vi "Text control 2 v6.4_pump-specific.vi"() -> ()   [LabVIEW 2016]
panel:
  in  "Tab Control":enum32{"Main", "Other parameters"}(tab)
  out "Line running":i32
  out "Total lines":i32
  out "Path":path=path "C:/users/rlp38/09Apr2009LTtesting/test2.txt"
  out "I vs Vg":cluster{"Y data in":dbl[], "X data in":dbl[]}[](graph)
  out "Is max":dbl format="%.2e"
  out "Id max":dbl format="%.2e"
  out "Ig max":dbl format="%.2e"
  out "Imax vs time":cluster{"Y data in":dbl[], "X data in":dbl[]}[](graph)
  out "Imin vs time":cluster{"Y data in":dbl[], "X data in":dbl[]}[](graph)
  out "I vs Vd":cluster{"Y data in":dbl[], "X data in":dbl[]}[](graph)
  in  "Script":string="#-------------------------------------------------------\n# SPM pump cleaning script\n#\n# Version: 0.5\n# Author: Dimitrios Simatos\n# Last updated: 2018-01-05\n#-------------------------------------------------------\n# Description\n#\n# This script is designed to run the cleaning sequence of the SPM OEM pump.\n# This script needs to be run 4 times!\n#-------------------------------------------------------\n# Changes\n#\n# Placed initialization and hard stop commands in the beginning.\n#-------------------------------------------------------\n# Important points\n#\n# Never leave any liquid in the pump to dry after the experiments. If they dry, the residue may block the valve.\n# Always run the cleaning cycle after the experiments.\n# Use clockwise rotation when going up in valve port numbers and vice versa.\n#-------------------------------------------------------\n# Things to do before running the script\n#\n# Set time units to minutes.\n# Set filenames.\n# Replace the tubing, if necessary.\n#-------------------------------------------------------\n# Port connections\n#\n# Port 1: Waste\n# Port 2: Waste\n# Port 3: Various cleaning liquids\n# Port 4: Waste\n# Port 5: Waste\n# Port 6: Waste\n#\n# Between each of the 4 runs, the settings of Port 3 will change, according to the cleaning protocol.\n# The settings for Port 3 are:\n# 1st run: 1% v/v solution of sodium hypochlorite in ultrapure water\n# 2nd run: 0.1% w/v solution of sodium dodecyl sulfate in ultrapure water\n# 3rd run: Ultrapure water\n# 4th run: Waste (in air, not immersed in liquid)\n#-------------------------------------------------------\n# Cleaning protocol for the SPM OEM pump (from the manual)\n#\n# A cleaning procedure should be performed at the end of each day or in between two different experiments.\n# An effective cleaning can be performed in the following manner:\n# • Bleach solution to kill microorganisms\n# 1. Prepare a solution of 1% chlorine bleach and deionized water\n#    NOTE: Prepare a 1% v/v solution of sodium hypochlorite in deionized water\n# 2. Prepare a reservoir and place 1 tubing in the bleach solution and 5 tubings in a waste recipient\n# 3. Pick up the bleach solution through 1 port to entirely fill the syringe\n# 4. Sequentially output the syringe content through the remaining ports and throw it to the waste\n# 5. Repeat operation at least 2 times\n# • Detergent solution to remove debris\n# 1. Prepare a solution of 0.1% detergent and deionized water\n#    NOTE: Prepare a 0.1% w/v solution of sodium dodecyl sulfate in deionized water\n# 2. Move the tubing from the bleach solution reservoir and place it into a reservoir of detergent solution\n# 3. Pick up the detergent solution through 1 port to entirely fill the syringe\n# 4. Sequentially output the detergent solution through the remaining ports into the waste recipient\n# 5. Repeat operation at least 2 times\n# • Rinsing water to prepare the pump for your next experiment\n# 1. Move the tubing from the detergent solution reservoir and place it into a reservoir of deionized water\n# 2. Pick up the rinsing solution through 1 port to entirely fill the syringe\n# 3. Sequentially output the rinse water through the remaining ports into the waste recipient\n# 4. Repeat operation at least 2 times\n# • Replace the tubing, if necessary\n#-------------------------------------------------------\n# Pumping cycles and execution time\n#\n# Execution time for a single cycle: 6 x (1 min + 10 sec) = 7 minutes\n# Total execution time: 4 x 7 = 28 minutes\n# Since the script has to run 4 times, the cleaning lasts for: 4 x 28 = 112 minutes\n# Air must be the last to be pumped through the valve, to remove all liquids.\n# There are 4 pumping cycles. Each one draws a different liquid through port 3 and pumps it sequentially through ports 1,2,4,5,6.\n# During the sequential pumping, each port receives 200 ml of liquid (20% of the total syringe volume = 600 \"plunger units\")\n# The device must be disconnected from the port during the cleaning procedure.\n# All cycles are similar, except cycle 1 has the initialization command uncommented and the first report valve command commented.\n#-------------------------------------------------------\n# Volume of liquid needed\n#\n# Volume of liquid needed per cycle: 1 ml\n# Total volume of liquid needed per script run: 4 x 1 = 4 ml\n# Since the script has to run 4 times, the first 3 with different liquids, I need:\n# 4 ml of 1% v/v solution of sodium hypochlorite in ultrapure water\n# 4 ml of 0.1% w/v solution of sodium dodecyl sulfate in ultrapure water\n# 4 ml of ultrapure water\n#-------------------------------------------------------\n# Parameters\n#\n# Syringe size: 1 ml\n# Step resolution N = 0.01 mm\n# Drawing flow V = 300 pulses/second (6000 ul/min)\n# Pumping flow V = 300 pulses/second (6000 ul/min)\n#-------------------------------------------------------\n# Pump initialization\npump /1T #hard stop pump\npump /1ZR #initialize pump\n#-------------------------------------------------------\n# Cycle 1\n# Fill the syringe\npump /1Q #query pump\npump /1? #report absolute plunger position\n#pump /1?6 #report valve position\nwait-min 1 #wait 1 minute\npump /1N0R #set step resolution: 0.01 mm\npump /1Q #query pump\npump /1? #report absolute plunger position (the plunger should be at 0)\npump /1?6 #report valve position\nwait 1000 #wait 1 second\npump /1V300R #choose speed: 300 steps/s (6000 ul/min)\npump /1Q #query pump\nwait 1000 #wait 1 second\npump /1I3R #go to port 3, clockwise rotation\npump /1Q #query pump\npump /1?6 #report valve position\nwait 1000 #wait 1 second\npump /1A3000R #go to absolute position 3000 (= draw 1 ml)\nwait 30000 #wait 30 seconds\npump /1Q #query pump\npump /1? #report absolute plunger position (the plunger should have finished moving)\n#pump /1?6 #report valve position\n# The sequential pumping begins\n# Port 1\npump /1O1R #switch to port 1, counterclockwise rotation\npump /1Q #query pump\npump /1?6 #report valve position\npump /1A2400R #go to absolute position 2400 (= pump 200 ul)\npump /1Q #query pump\npump /1? #report absolute plunger position (the plunger should be moving to 0)\nwait-min 1 #wait 1 minute\npump /1? #report absolute plunger position (the plunger should have finished moving)\n# Port 2\npump /1I2R #switch to port 2, clockwise rotation\npump /1Q #query pump\npump /1?6 #report valve position\npump /1A1800R #go to absolute position 1800 (= pump 200 ul)\npump /1Q #query pump\npump /1? #report absolute plunger position (the plunger should be moving to 0)\nwait-min 1 #wait 1 minute\npump /1? #report absolute plunger position (the plunger should have finished moving)\n# Port 4\npump /1I4R #switch to port 4, clockwise rotation\npump /1Q #query pump\npump /1?6 #report valve position\npump /1A1200R #go to absolute position 1200 (= pump 200 ul)\npump /1Q #query pump\npump /1? #report absolute plunger position (the plunger should be moving to 0)\nwait-min 1 #wait 1 minute\npump /1? #report absolute plunger position (the plunger should have finished moving)\n# Port 5\npump /1I5R #switch to port 5, clockwise rotation\npump /1Q #query pump\npump /1?6 #report valve position\npump /1A600R #go to absolute position 600 (= pump 200 ul)\npump /1Q #query pump\npump /1? #report absolute plunger position (the plunger should be moving to 0)\nwait-min 1 #wait 1 minute\npump /1? #report absolute plunger position (the plunger should have finished moving)\n# Port 6\npump /1I6R #switch to port 6, clockwise rotation\npump /1Q #query pump\npump /1?6 #report valve position\npump /1A0R #go to absolute position 0 (= pump 200 ul)\npump /1Q #query pump\npump /1? #report absolute plunger position (the plunger should be moving to 0)\nwait-min 1 #wait 1 minute\npump /1? #report absolute plunger position (the plunger should have finished moving)\n#-------------------------------------------------------\n# Cycle 2\n# Fill the syringe\n#pump /1ZR #initialize pump\npump /1Q #query pump\npump /1? #report absolute plunger position\npump /1?6 #report valve position\nwait-min 1 #wait 1 minute\npump /1N0R #set step resolution: 0.01 mm\npump /1Q #query pump\npump /1? #report absolute plunger position (the plunger should be at 0)\npump /1?6 #report valve position\nwait 1000 #wait 1 second\npump /1V300R #choose speed: 300 steps/s (6000 ul/min)\npump /1Q #query pump\nwait 1000 #wait 1 second\npump /1O3R #go to port 3, counterclockwise rotation\npump /1Q #query pump\npump /1?6 #report valve position\nwait 1000 #wait 1 second\npump /1A3000R #go to absolute position 3000 (= draw 1 ml)\nwait 30000 #wait 30 seconds\npump /1Q #query pump\npump /1? #report absolute plunger position (the plunger should have finished moving)\n#pump /1?6 #report valve position\n# The sequential pumping begins\n# Port 1\npump /1O1R #switch to port 1, counterclockwise rotation\npump /1Q #query pump\npump /1?6 #report valve position\npump /1A2400R #go to absolute position 2400 (= pump 200 ul)\npump /1Q #query pump\npump /1? #report absolute plunger position (the plunger should be moving to 0)\nwait-min 1 #wait 1 minute\npump /1? #report absolute plunger position (the plunger should have finished moving)\n# Port 2\npump /1I2R #switch to port 2, clockwise rotation\npump /1Q #query pump\npump /1?6 #report valve position\npump /1A1800R #go to absolute position 1800 (= pump 200 ul)\npump /1Q #query pump\npump /1? #report absolute plunger position (the plunger should be moving to 0)\nwait-min 1 #wait 1 minute\npump /1? #report absolute plunger position (the plunger should have finished moving)\n# Port 4\npump /1I4R #switch to port 4, clockwise rotation\npump /1Q #query pump\npump /1?6 #report valve position\npump /1A1200R #go to absolute position 1200 (= pump 200 ul)\npump /1Q #query pump\npump /1? #report absolute plunger position (the plunger should be moving to 0)\nwait-min 1 #wait 1 minute\npump /1? #report absolute plunger position (the plunger should have finished moving)\n# Port 5\npump /1I5R #switch to port 5, clockwise rotation\npump /1Q #query pump\npump /1?6 #report valve position\npump /1A600R #go to absolute position 600 (= pump 200 ul)\npump /1Q #query pump\npump /1? #report absolute plunger position (the plunger should be moving to 0)\nwait-min 1 #wait 1 minute\npump /1? #report absolute plunger position (the plunger should have finished moving)\n# Port 6\npump /1I6R #switch to port 6, clockwise rotation\npump /1Q #query pump\npump /1?6 #report valve position\npump /1A0R #go to absolute position 0 (= pump 200 ul)\npump /1Q #query pump\npump /1? #report absolute plunger position (the plunger should be moving to 0)\nwait-min 1 #wait 1 minute\npump /1? #report absolute plunger position (the plunger should have finished moving)\n#-------------------------------------------------------\n# Cycle 3\n# Fill the syringe\n#pump /1ZR #initialize pump\npump /1Q #query pump\npump /1? #report absolute plunger position\npump /1?6 #report valve position\nwait-min 1 #wait 1 minute\npump /1N0R #set step resolution: 0.01 mm\npump /1Q #query pump\npump /1? #report absolute plunger position (the plunger should be at 0)\npump /1?6 #report valve position\nwait 1000 #wait 1 second\npump /1V300R #choose speed: 300 steps/s (6000 ul/min)\npump /1Q #query pump\nwait 1000 #wait 1 second\npump /1O3R #go to port 3, counterclockwise rotation\npump /1Q #query pump\npump /1?6 #report valve position\nwait 1000 #wait 1 second\npump /1A3000R #go to absolute position 3000 (= draw 1 ml)\nwait 30000 #wait 30 seconds\npump /1Q #query pump\npump /1? #report absolute plunger position (the plunger should have finished moving)\n#pump /1?6 #report valve position\n# The sequential pumping begins\n# Port 1\npump /1O1R #switch to port 1, counterclockwise rotation\npump /1Q #query pump\npump /1?6 #report valve position\npump /1A2400R #go to absolute position 2400 (= pump 200 ul)\npump /1Q #query pump\npump /1? #report absolute plunger position (the plunger should be moving to 0)\nwait-min 1 #wait 1 minute\npump /1? #report absolute plunger position (the plunger should have finished moving)\n# Port 2\npump /1I2R #switch to port 2, clockwise rotation\npump /1Q #query pump\npump /1?6 #report valve position\npump /1A1800R #go to absolute position 1800 (= pump 200 ul)\npump /1Q #query pump\npump /1? #report absolute plunger position (the plunger should be moving to 0)\nwait-min 1 #wait 1 minute\npump /1? #report absolute plunger position (the plunger should have finished moving)\n# Port 4\npump /1I4R #switch to port 4, clockwise rotation\npump /1Q #query pump\npump /1?6 #report valve position\npump /1A1200R #go to absolute position 1200 (= pump 200 ul)\npump /1Q #query pump\npump /1? #report absolute plunger position (the plunger should be moving to 0)\nwait-min 1 #wait 1 minute\npump /1? #report absolute plunger position (the plunger should have finished moving)\n# Port 5\npump /1I5R #switch to port 5, clockwise rotation\npump /1Q #query pump\npump /1?6 #report valve position\npump /1A600R #go to absolute position 600 (= pump 200 ul)\npump /1Q #query pump\npump /1? #report absolute plunger position (the plunger should be moving to 0)\nwait-min 1 #wait 1 minute\npump /1? #report absolute plunger position (the plunger should have finished moving)\n# Port 6\npump /1I6R #switch to port 6, clockwise rotation\npump /1Q #query pump\npump /1?6 #report valve position\npump /1A0R #go to absolute position 0 (= pump 200 ul)\npump /1Q #query pump\npump /1? #report absolute plunger position (the plunger should be moving to 0)\nwait-min 1 #wait 1 minute\npump /1? #report absolute plunger position (the plunger should have finished moving)\n#-------------------------------------------------------\n# Cycle 4\n# Fill the syringe\n#pump /1ZR #initialize pump\npump /1Q #query pump\npump /1? #report absolute plunger position\npump /1?6 #report valve position\nwait-min 1 #wait 1 minute\npump /1N0R #set step resolution: 0.01 mm\npump /1Q #query pump\npump /1? #report absolute plunger position (the plunger should be at 0)\npump /1?6 #report valve position\nwait 1000 #wait 1 second\npump /1V300R #choose speed: 300 steps/s (6000 ul/min)\npump /1Q #query pump\nwait 1000 #wait 1 second\npump /1O3R #go to port 3, counterclockwise rotation\npump /1Q #query pump\npump /1?6 #report valve position\nwait 1000 #wait 1 second\npump /1A3000R #go to absolute position 3000 (= draw 1 ml)\nwait 30000 #wait 30 seconds\npump /1Q #query pump\npump /1? #report absolute plunger position (the plunger should have finished moving)\n#pump /1?6 #report valve position\n# The sequential pumping begins\n# Port 1\npump /1O1R #switch to port 1, counterclockwise rotation\npump /1Q #query pump\npump /1?6 #report valve position\npump /1A2400R #go to absolute position 2400 (= pump 200 ul)\npump /1Q #query pump\npump /1? #report absolute plunger position (the plunger should be moving to 0)\nwait-min 1 #wait 1 minute\npump /1? #report absolute plunger position (the plunger should have finished moving)\n# Port 2\npump /1I2R #switch to port 2, clockwise rotation\npump /1Q #query pump\npump /1?6 #report valve position\npump /1A1800R #go to absolute position 1800 (= pump 200 ul)\npump /1Q #query pump\npump /1? #report absolute plunger position (the plunger should be moving to 0)\nwait-min 1 #wait 1 minute\npump /1? #report absolute plunger position (the plunger should have finished moving)\n# Port 4\npump /1I4R #switch to port 4, clockwise rotation\npump /1Q #query pump\npump /1?6 #report valve position\npump /1A1200R #go to absolute position 1200 (= pump 200 ul)\npump /1Q #query pump\npump /1? #report absolute plunger position (the plunger should be moving to 0)\nwait-min 1 #wait 1 minute\npump /1? #report absolute plunger position (the plunger should have finished moving)\n# Port 5\npump /1I5R #switch to port 5, clockwise rotation\npump /1Q #query pump\npump /1?6 #report valve position\npump /1A600R #go to absolute position 600 (= pump 200 ul)\npump /1Q #query pump\npump /1? #report absolute plunger position (the plunger should be moving to 0)\nwait-min 1 #wait 1 minute\npump /1? #report absolute plunger position (the plunger should have finished moving)\n# Port 6\npump /1I6R #switch to port 6, clockwise rotation\npump /1Q #query pump\npump /1?6 #report valve position\npump /1A0R #go to absolute position 0 (= pump 200 ul)\npump /1Q #query pump\npump /1? #report absolute plunger position (the plunger should be moving to 0)\nwait-min 1 #wait 1 minute\npump /1? #report absolute plunger position (the plunger should have finished moving)\n#-------------------------------------------------------"
  out "Command running:":string
  out "Serial port data":string
  out "Elapsed Time":dbl caption="Elapsed Time (s)"
  in  "Time Units":u16(ring)=1 items=["Seconds", "Minutes", "Hours"]
  in  "Time Offset":dbl caption="Set Start Time (s)"
  in  "Reset":bool
  in  "Auto Reset":bool
  in  "integration time":u32(slide) max=2 step=1 scale=0.0..2.0
  in  "Interrupt scan":bool
  out "Absolute plunger position vs time":cluster{"Y data in":dbl[], "X data in":dbl[]}[](graph)
  out "Valve position vs time":cluster{"Y data in":dbl[], "X data in":dbl[]}[](graph)
  out "Is on":dbl format="%.2e"
  out "Id on":dbl format="%.2e"
  out "Ig on":dbl format="%.2e"
  out "Ion vs time":cluster{"Y data in":dbl[], "X data in":dbl[]}[](graph)
  out "Ioff vs time":cluster{"Y data in":dbl[], "X data in":dbl[]}[](graph)
  out "Ig min":dbl format="%.2e"
  out "Id min":dbl format="%.2e"
  out "Is min":dbl format="%.2e"
  out "Is off":dbl format="%.2e"
  out "Id off":dbl format="%.2e"
  out "Ig off":dbl format="%.2e"
  in  "Integration time (long)":dbl=0.32 min=0.04 max=2.0 step=0.02 format="%.2f"
  in  "Integration time (short)":dbl=0.0019 min=8e-05 max=0.0019 step=8e-05 format="%^.0e"
  in  "Gate: Compliance":dbl=0.001 format="%.8f"
  in  "Drain: Compliance":dbl=0.001 format="%.8f"
  in  "Hard stop pump":bool
  in  "Halt pump":bool
  in  "Interrupt program":bool
  in  "Suffix (script)":string="step_1_up-H2O_initial_script.txt"
  in  "Filename (variable part)":string="step_1_up-H2O_initial_"
  in  "Plot output curve extrema vs time":bool
  in  "Plot transfer curve extrema vs time":bool=TRUE
  in  "Gate Range\nmode":u16(ring) items=["Auto", "Limited", "Fixed"]
  in  "Gate Range":u8(slide)=6 max=11 scale=0.0..11.0
  in  "Source/Drain\nRange mode":u16(ring) items=["Auto", "Limited", "Fixed"]
  in  "Source/Drain Range":u8(slide)=6 max=11 scale=0.0..11.0
  in  "Panel Controls":T1={"Emergency Stop"=refnum, "TransGraph Max"=1e-05, "Text/Graph (text=false)"=TRUE} {"TransGraph Max" format="%.2e"}
  in  "Panel Controls 2":T2={"Emergency Stop"=refnum, "TransGraph Max"=1e-05, "Text/Graph (text=false)"=TRUE, "TransGraph Min"=1e-11} {"TransGraph Min" format="%.2e"; "TransGraph Max" format="%.2e"}
  in  "SMU4":cluster{"on/off":bool, "Voltage":dbl} {"Voltage" min=-100.0 max=100.0 format="%.2f"}
  in  "Full Reset":bool
  in  "Standby":T3
  out "error out":errorcluster
  in  "Delay before read (ms)":u32=1000
  in  "byte count":u32=64
  in  "Serial End Mode for Reads":u16(ring)=2 items=["None", "LastBit", "TermChar"]
  in  "Timeout (ms)":u32=10000
  in  "Enable Termination\nChar (T)":bool=TRUE
  in  "Termination char\n(0xA = '\\n' = LF)\n(0xD = '\\r' = CR)":u8=13 format="%.0x"
  in  "flow control":u16(ring) items=["None"=0, "XON/XOFF"=1, "RTS/CTS"=2, "DTR/DSR"=4]
  in  "stop bits":u16(ring)=10 items=["1.0"=10, "1.5"=15, "2.0"=20]
  in  "parity":u16(ring) items=["None", "Odd", "Even", "Mark", "Space"]
  in  "data bits":u16=8 min=5 max=8 step=1
  in  "VISA resource name":refnum<visa-resource-name>="COM6"
  in  "baud rate":u32=9600
  out "Timings Indicator":T4
  in  "Timings (overwritten by the Front Panel)":T5={"integration time"=0, "Short/Long integration time"=0.00064, "hold time (sec)"=0.0, "delay time (sec)"=0.0, "Step Time (0 disables)"=0.0, "sweep method"=0, "Pulse period"=0.005, "Base voltage"=0.0, "Pulse width"=0.0005} {"Pulse width" min=0.0005 max=0.1 step=0.0001 format="%.4f"; "Base voltage" format="%^.4e"; "Pulse period" min=0.005 max=1.0 step=0.0001 format="%.4f"; "sweep method" items=["Continuous", "Pulsed"]; "Step Time (0 disables)" format="%.2f"; "delay time (sec)" format="%.4f"; "hold time (sec)" format="%.4f"; "Short/Long integration time" format="%^.0e"; "integration time" scale=0.0..2.0}
  in  "Gate":T6={"Gate Start"=0.0, "Gate Stop"=2.0, "Gate Step (linear only)"=1.0, "Gate Compliance"=0.0001, "Gate PComp"=0.0, "Range mode"=0, "Range"=6} {"Range" max=11 scale=0.0..11.0; "Range mode" items=["Auto", "Limited", "Fixed"]; "Gate PComp" format="%^.2e"; "Gate Compliance" format="%^.2e"; "Gate Step (linear only)" format="%^.4e"; "Gate Stop" format="%^.4e"; "Gate Start" format="%^.4e"}
  in  "Drain 2":T7={"Drain Start"=0.0, "Drain Stop"=2.0, "Drain Compliance"=0.0001, "Drain Step"=1.0, "Drain PComp"=0.0, "Range mode"=0, "Range"=6} {"Range" max=11 scale=0.0..11.0; "Range mode" items=["Auto", "Limited", "Fixed"]; "Drain PComp" format="%^.2e"; "Drain Step" format="%^.4e"; "Drain Compliance" format="%^.2e"; "Drain Stop" format="%^.4e"; "Drain Start" format="%^.4e"}
  # "Syntax:\nitime [s|m|l] time(sec): [s|m|l] determines the integration time setting (small|medium|long) and time sets the value.\nNOTE: The value of the integration time has to be within the range allowed by its category (s|m|l), otherwise, the closest value will be used. (e.g. if the category is set to short but the time value is very long, the actual value used will be the maximum short integration time.\nIntegration times:\n    Short: Default: 640 us. Range: 8E-5 - 1.92E-3 seconds.\n    Medium: Fixed at 1 NPL cycle (0.02 seconds).\n    Long: Default: 16 NPL cycles (0.32 seconds). Range: 2-100 NPL cycles (0.04 seconds - 2 seconds).\ngaterangemode [a|l|f]\ndrainrangemode [a|l|f]\npulsed [on|off] PulsePeriod(sec) PulseBaseVoltage PulseONWidth(sec)\nstandby [on l off]\nwait NumMilliseconds\nwait-min NumMinutes\n# texthere = comment\ntransfer [s|d] VgStart VgStop VgStep VdStart VdStop VdStep\noutput [s|d] VgStart VgStop VgStep VdStart VdStop VdStep\nsample Vg Vd NumSamples Time(s) SampleInterval(s)\nsamplei Idg NumSamples Time(s) SampleInterval(s) VDGcompliance\n100 samples is approximately 13 seconds with medium integration\n# if in doubt use SampleInterval(s) = 0.004\nstressV VG VD IGcompliance IDcompliance Duration(sec)\nstressI IDG VDGcompliance Duration(sec)\nvsu2pulse Bias Duration(s)\npulsedstressV [s|d] VEstop VgON VgOFF Period(s) PulseONwidth(s) Vd\nsample-fpp Vg Vd NumSamples Time\nresample-fpp Vg Vd\ntransfer-fpp [s|d] VgStart VgStop VgStep VdStart VdStop VdStep\noutput-fpp [s|d] VgStart VgStop VgStep VdStart VdStop VdStep\nserial SerialPortCommand\npump SerialPortCommand for the SPM pump\n\nSPM Pump Syntax (<x>: pump number, use 1 if only one pump):\nif the command syntax contains [R], then append the letter R to the command\n/<x>Q: query (a query command should follow each command)\n/<x>Z[R] or /<x>Y[R]: initialize pump\n/<x>N<n>[R] (<n>=0,1): <0> (<1>) microstep 0.01 mm (0.00125 mm) resolution\n/<x>I<n> (<n>=0-6): turn to port number n (clockwise)\n/<x>O<n> (<n>=0-6): turn to port number n (counterclockwise)\n/<x>X: Re-execute last command string\n/<x>G<n>[R] (<n>=0-60000): repeat command sequence (default: 0, 0=loop forever)\n/<x>g: Mark the start of a repeat sequence (max = 10)\n/<x>M<n>[R] (<n>=0-86400000): delay command execution by n milliseconds\n/<x>H: Halt; Pause the sequence after finishing the current move\n/<x>T: Hardstop; Interrupt the current move and suppress it from the sequence\n/<x>A<n>[R] (<n>=0-3000 with N=0, 0-24000 with N=1): absolute position\n/<x>P<n>[R] (<n>=0-3000 with N=0, 0-24000 with N=1): relative pickup\n/<x>D<n>[R] (<n>=0-3000 with N=0, 0-24000 with N=1): relative dispense\n/<x>V<n>[R] (<n>=1-1600 default: 150): set peak speed (pulses/sec)\nNOTE: The lowest speed limit is 1 pulse/sec, not 5, as the manual states.\n/<x>S<n>[R] (<n>=10-40 default: 22): set speed (NOT in pulses/sec, look in manual)\nNOTE: When controlled with absolute position, one does not need to pay special attention to the syringe that is mounted on the pump.\nWithdraw from lower stage (ports 3, 5), dispense from higher stage (ports 2, 4, 6).\nConnect Port 1 to waste."
  # "Time"
  # "1\n2\n3\n4\n5\n6\n7\n8\n9\n10\n11\n12\n13\n14\n15\n16\n17\n18\n19\n20"
  # "Serial port settings"
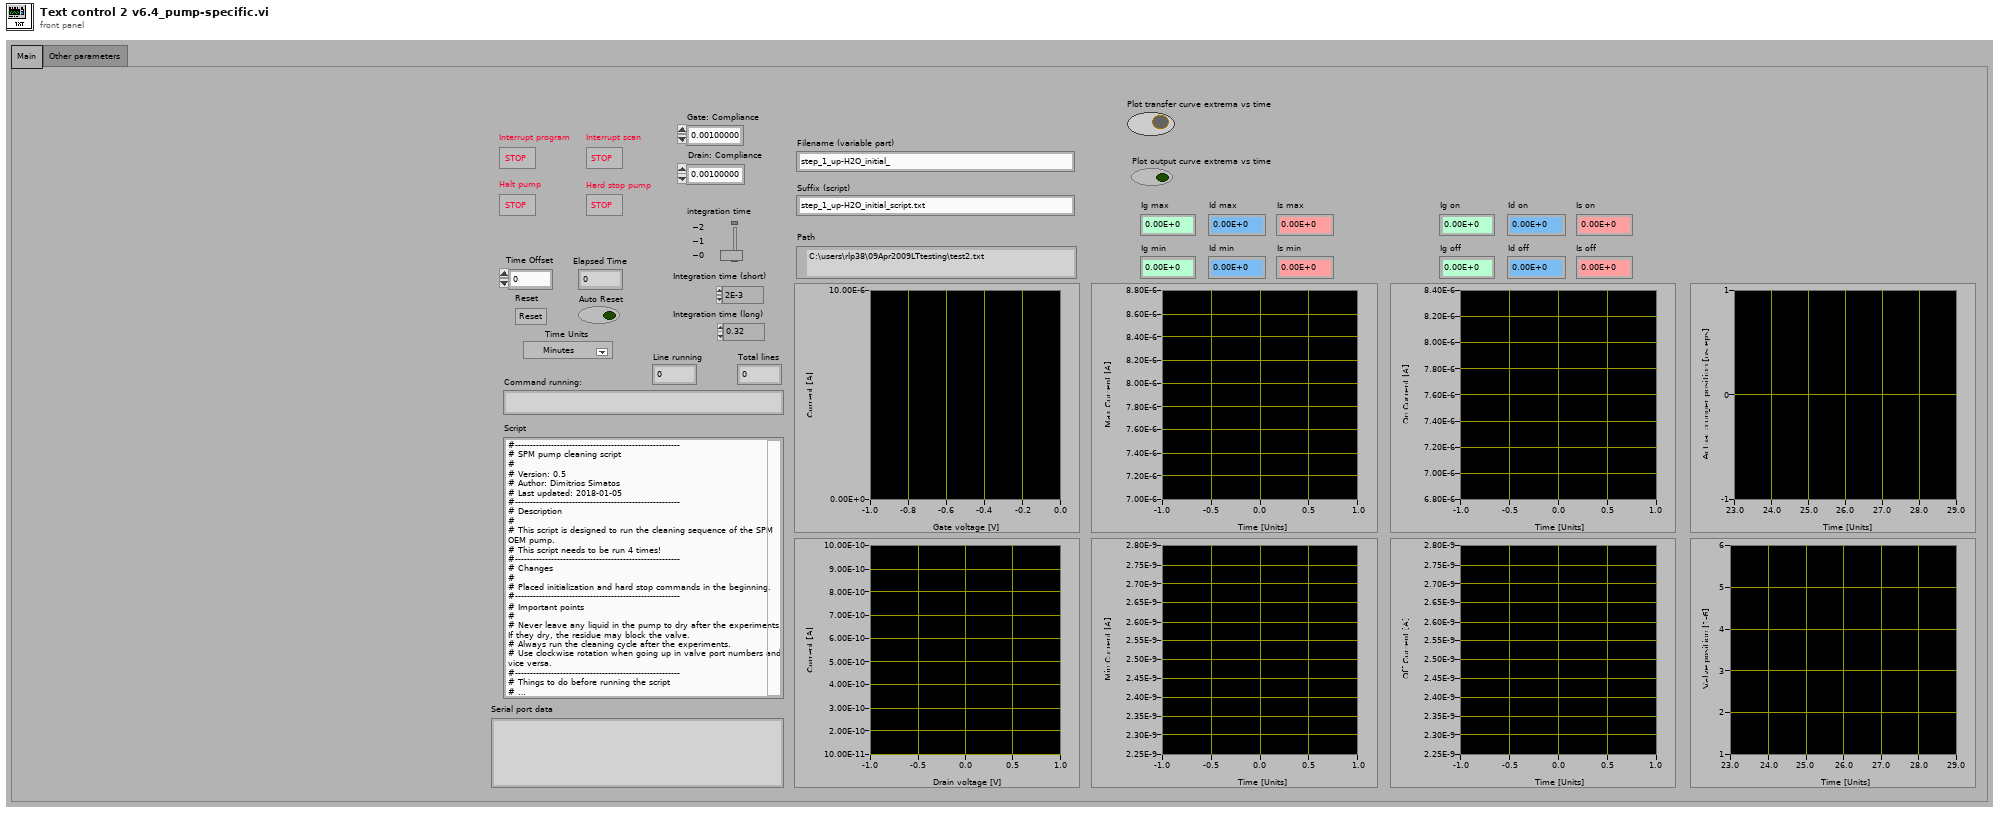
[diagram p1: front panel]
types:
  T1 = cluster{"Emergency Stop":refnum<vi>, "TransGraph Max":dbl, "Text/Graph (text=false)":bool}
  T2 = cluster{"Emergency Stop":refnum<vi>, "TransGraph Max":dbl, "Text/Graph (text=false)":bool, "TransGraph Min":dbl}
  T3 = cluster{"Gate Standby":bool, "Drain Standby":bool}
  T4 = cluster{"integration time (0:s, 1:m, 2:l)":u32, "Short/Long integration time":dbl, "hold time (sec)":dbl, "delay time (sec)":dbl, "Step Time (0 disables)":dbl, "sweep method":u16, "Pulse period":dbl, "Base voltage":dbl, "Pulse width":dbl}
  T5 = cluster{"integration time":u32, "Short/Long integration time":dbl, "hold time (sec)":dbl, "delay time (sec)":dbl, "Step Time (0 disables)":dbl, "sweep method":u16, "Pulse period":dbl, "Base voltage":dbl, "Pulse width":dbl}
  T6 = cluster{"Gate Start":dbl, "Gate Stop":dbl, "Gate Step (linear only)":dbl, "Gate Compliance":dbl, "Gate PComp":dbl, "Range mode":u16, "Range":u8}
  T7 = cluster{"Drain Start":dbl, "Drain Stop":dbl, "Drain Compliance":dbl, "Drain Step":dbl, "Drain PComp":dbl, "Range mode":u16, "Range":u8}
  T8 = enum16{"open", "replace", "create", "open or create", "replace or create", "replace or create with confirmation"}
  T9 = cluster{"V2 Start":dbl, "V2 Step":dbl, "Number of points":i32}
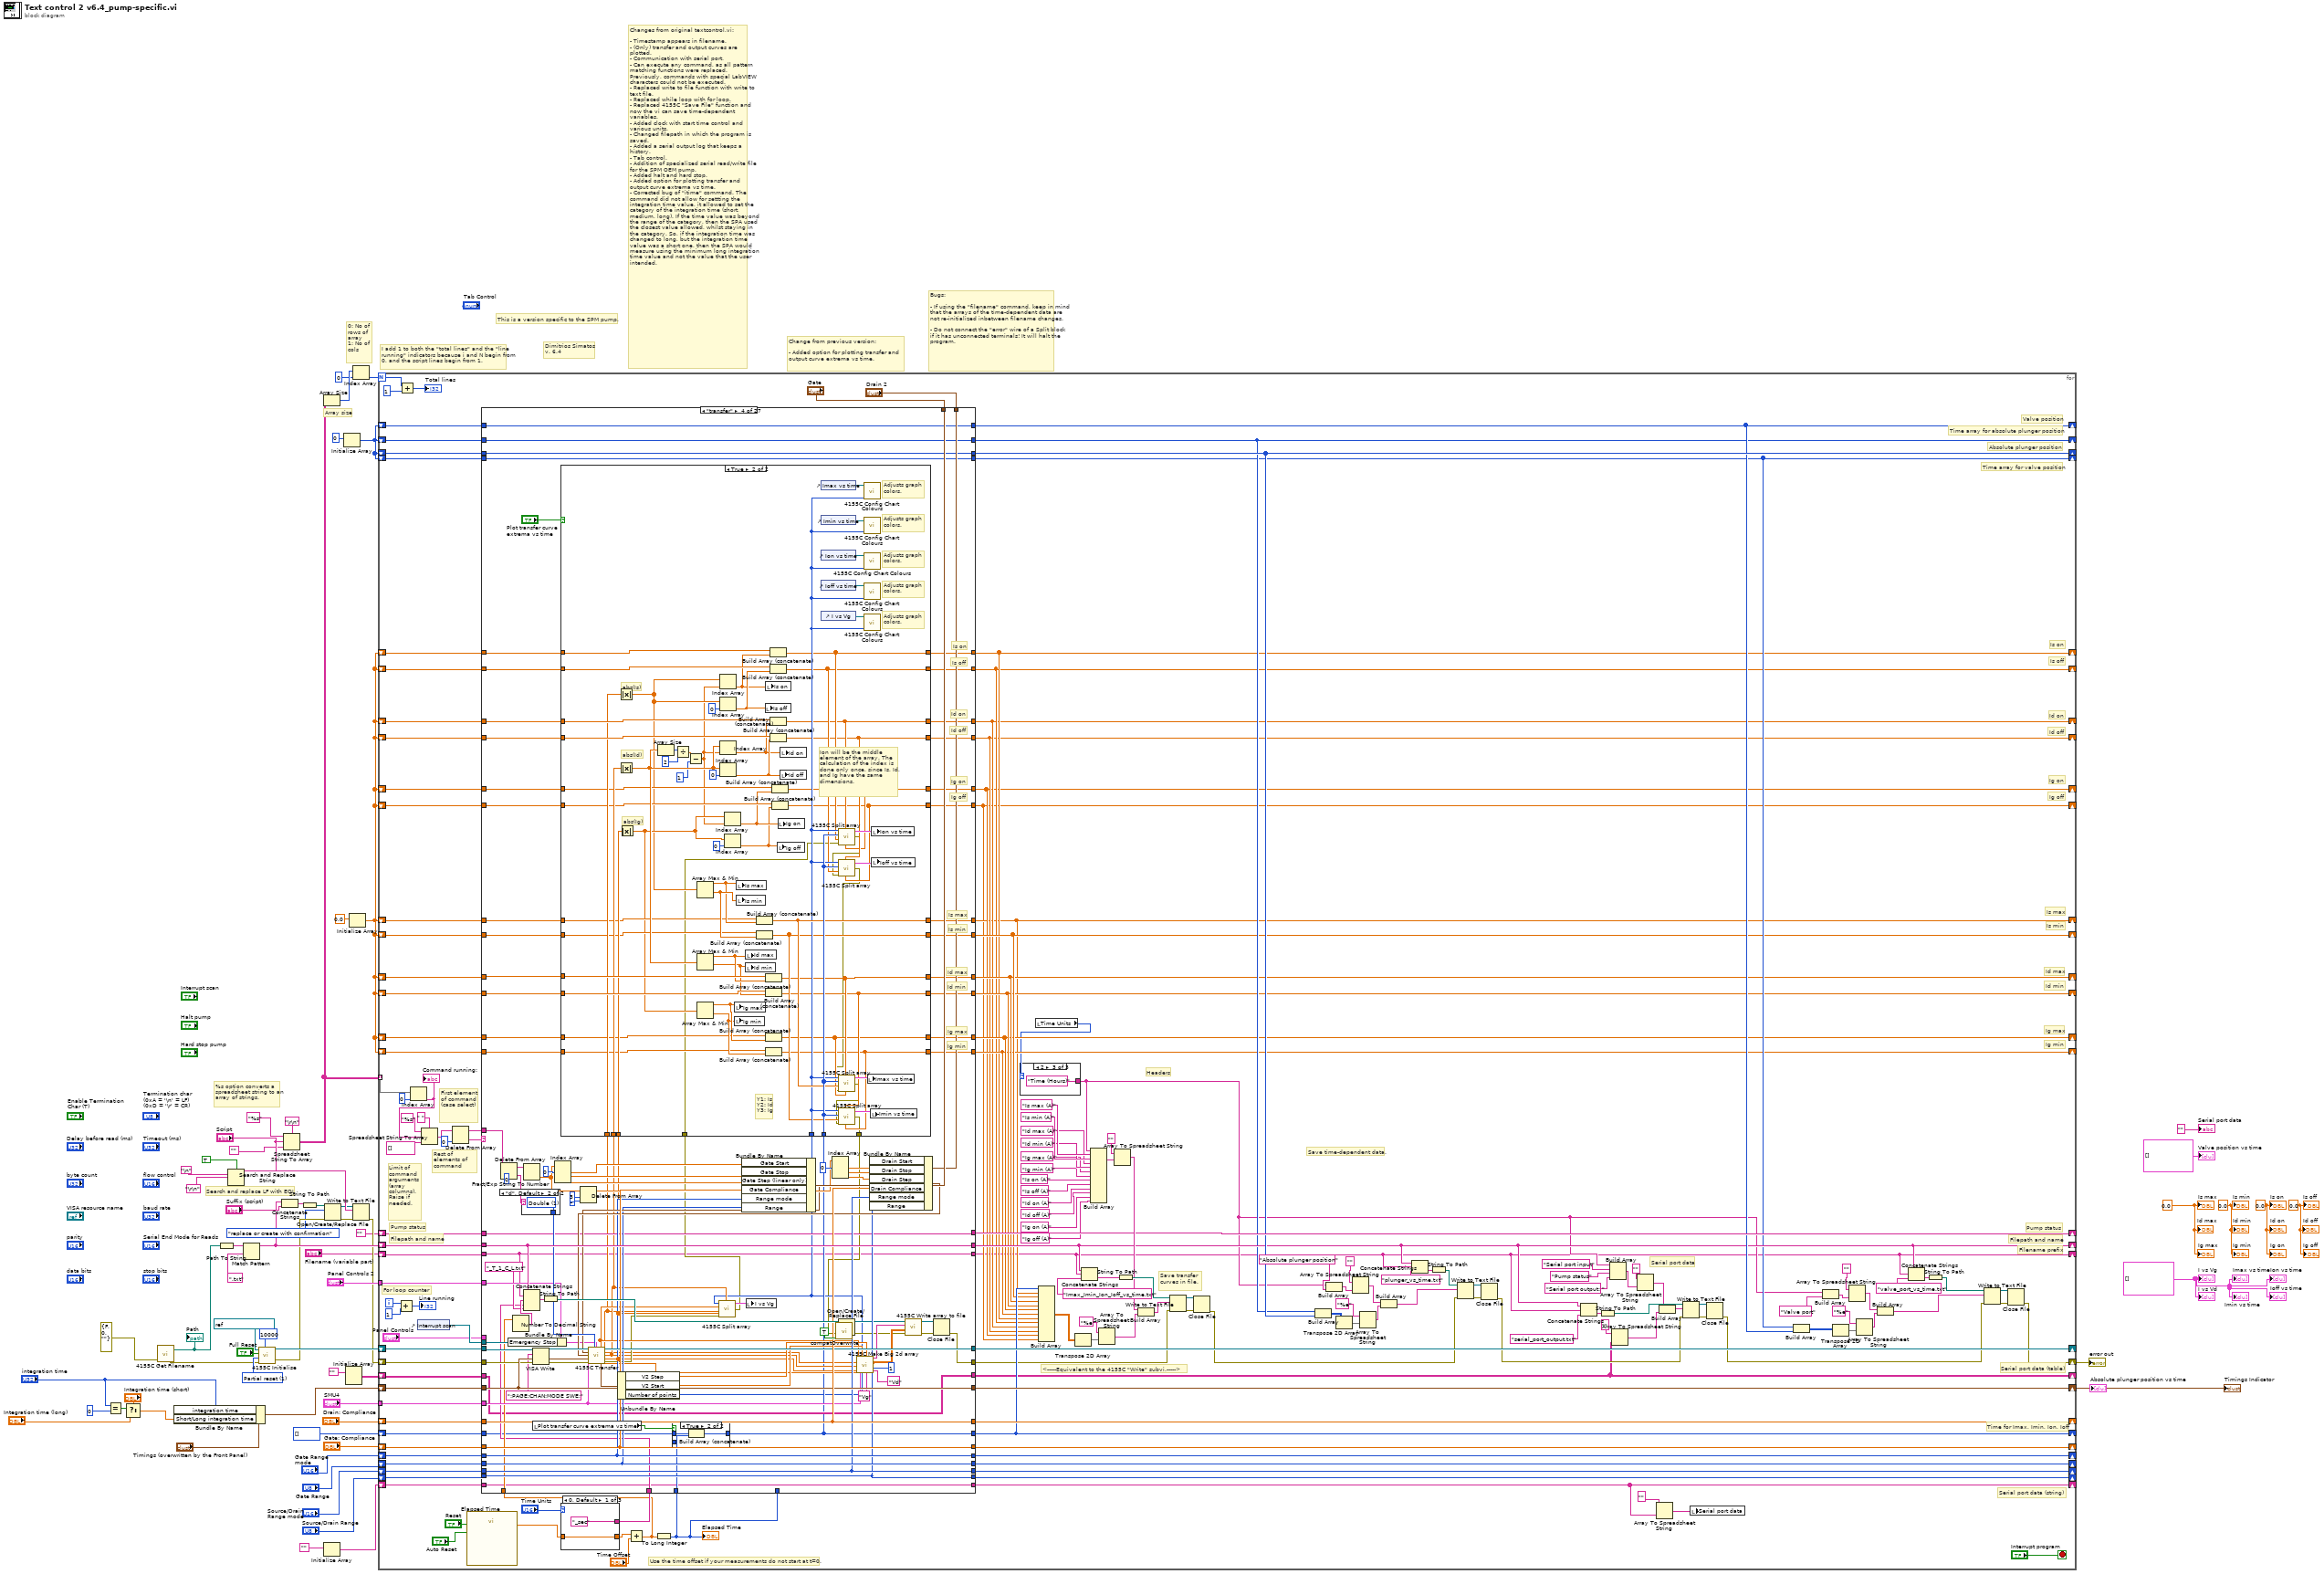
[diagram p0: block diagram]
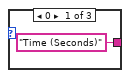
[diagram p2: hidden frame]
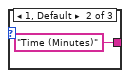
[diagram p3: hidden frame]
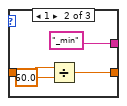
[diagram p4: hidden frame]
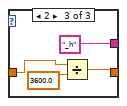
[diagram p5: hidden frame]
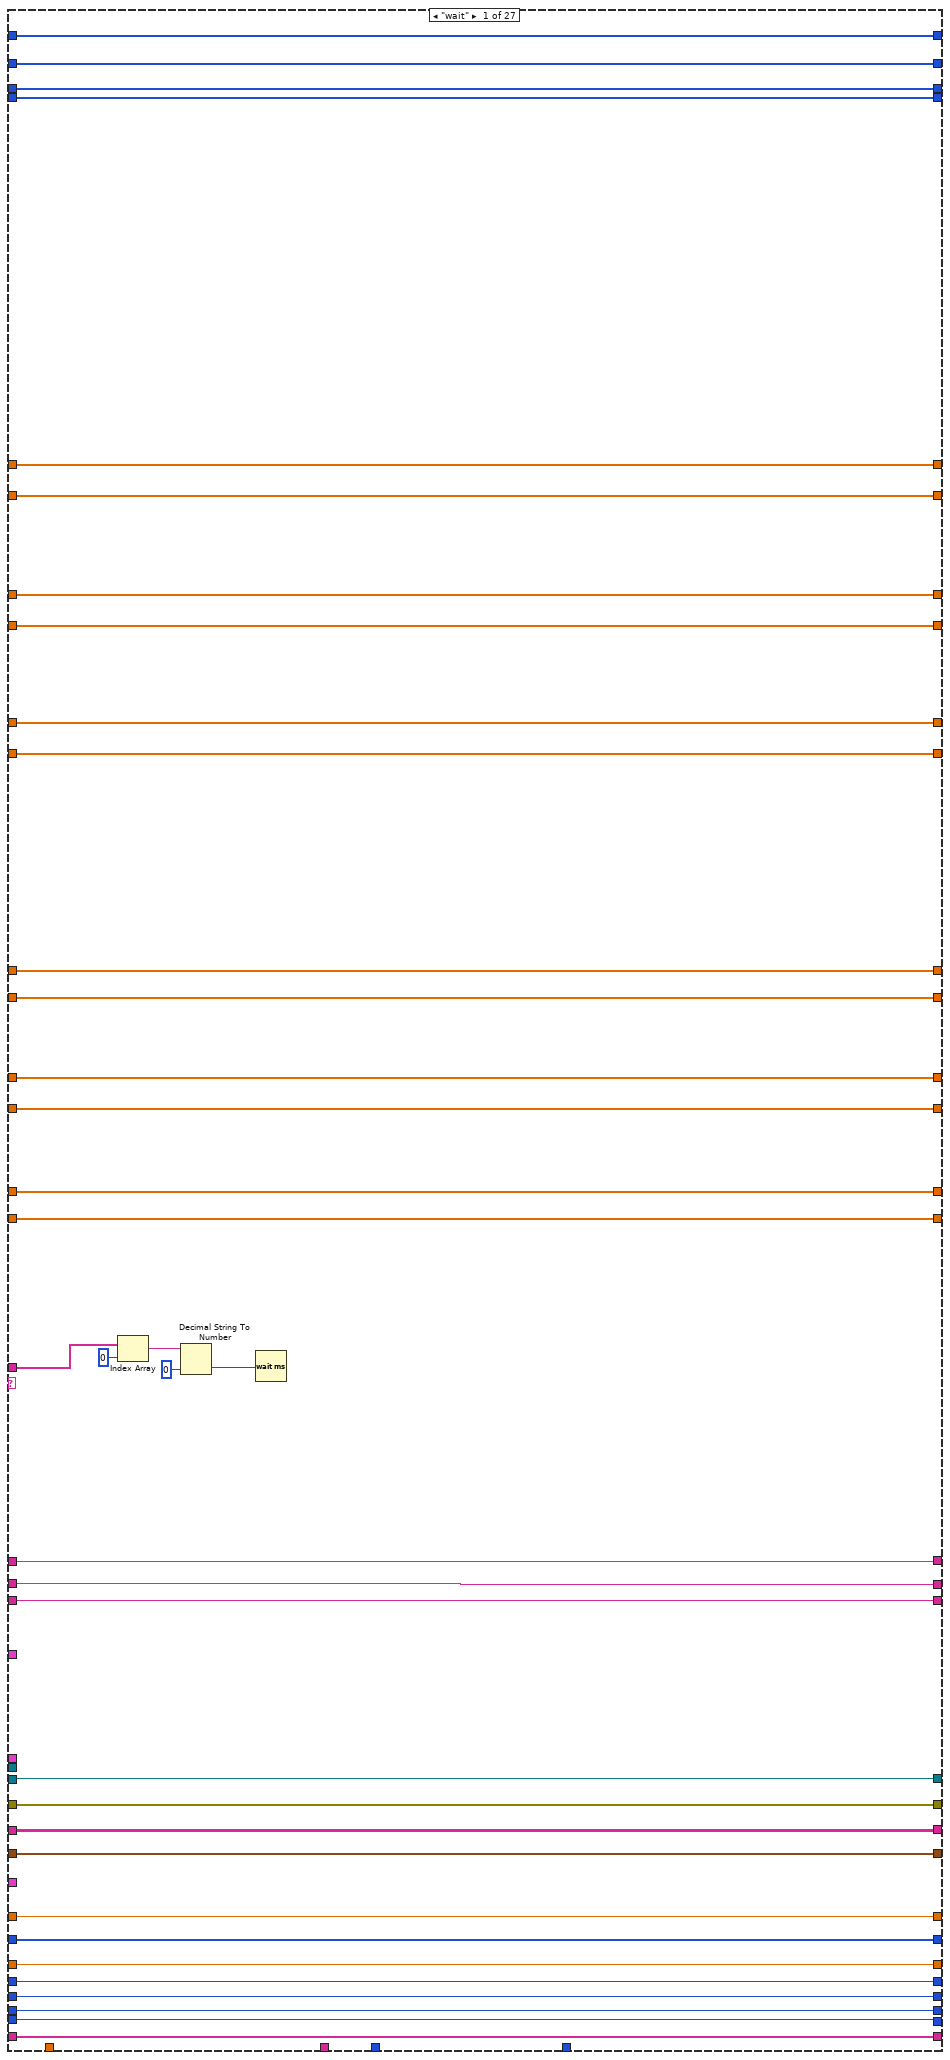
[diagram p6: hidden frame]
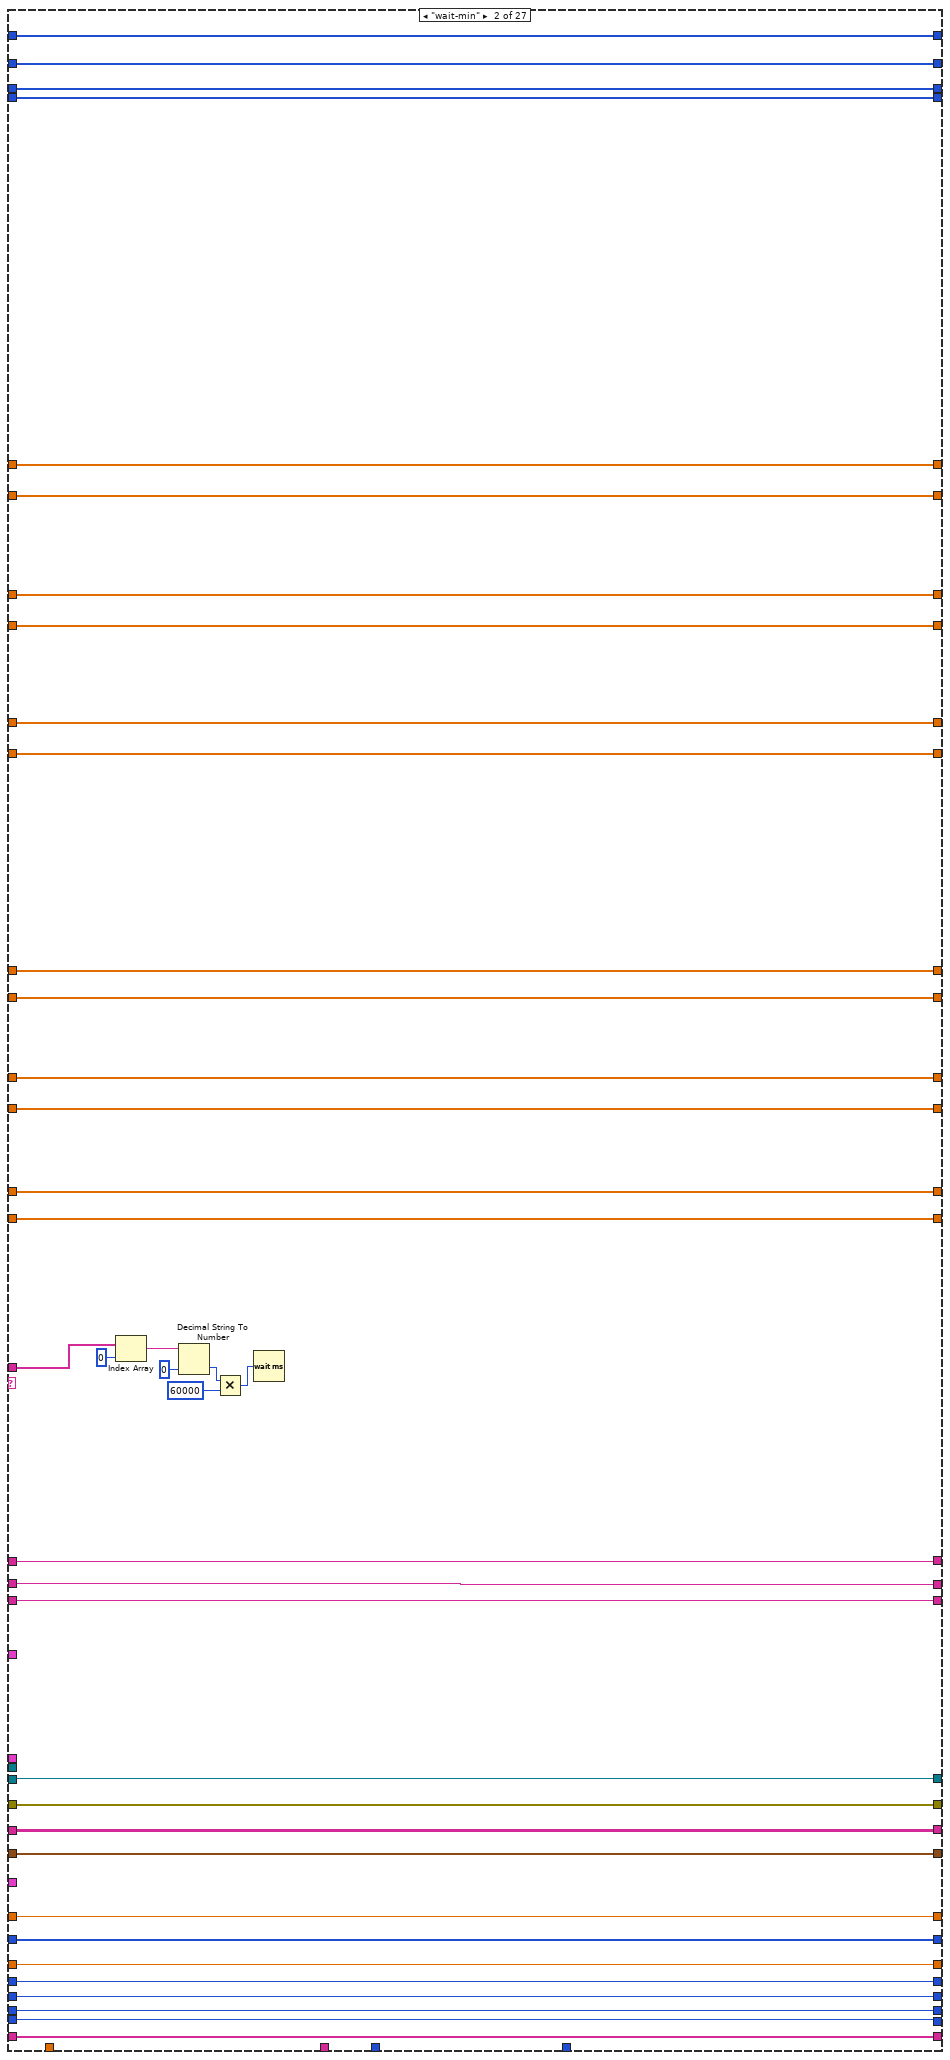
[diagram p7: hidden frame]
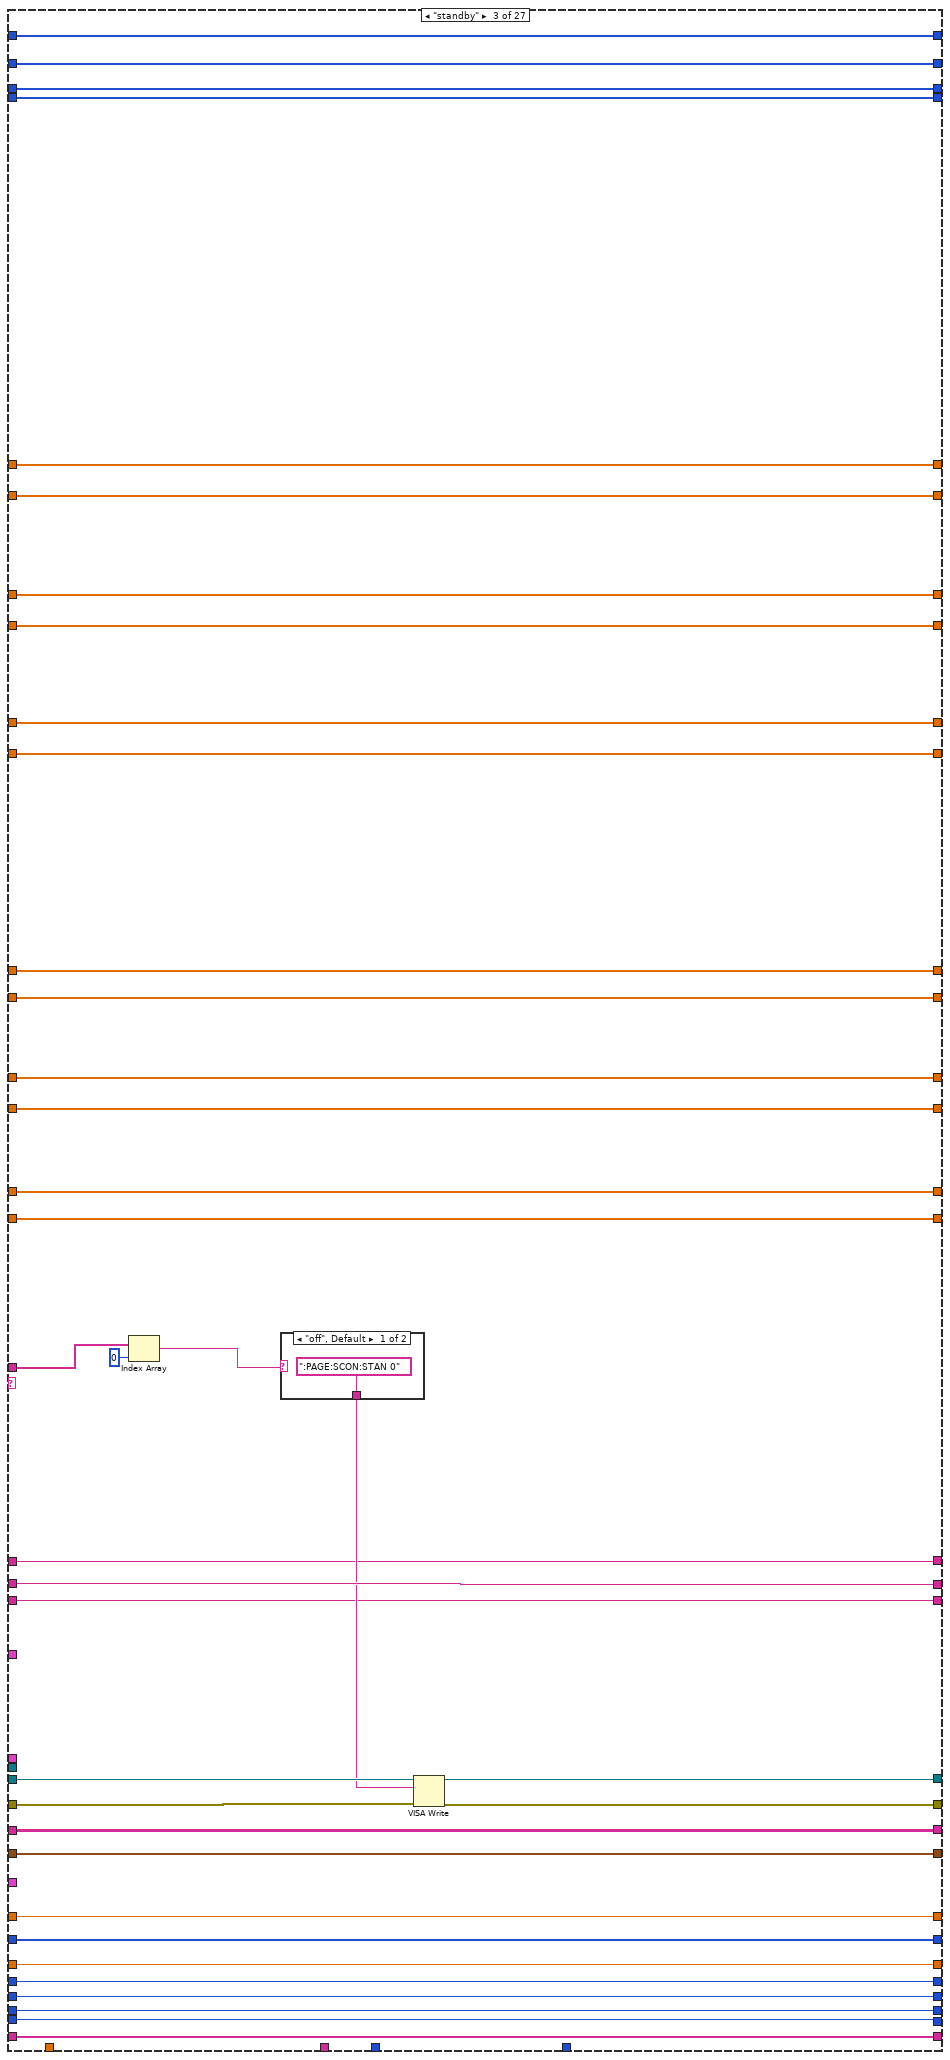
[diagram p8: hidden frame]
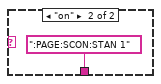
[diagram p9: hidden frame]
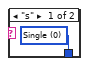
[diagram p12: hidden frame]
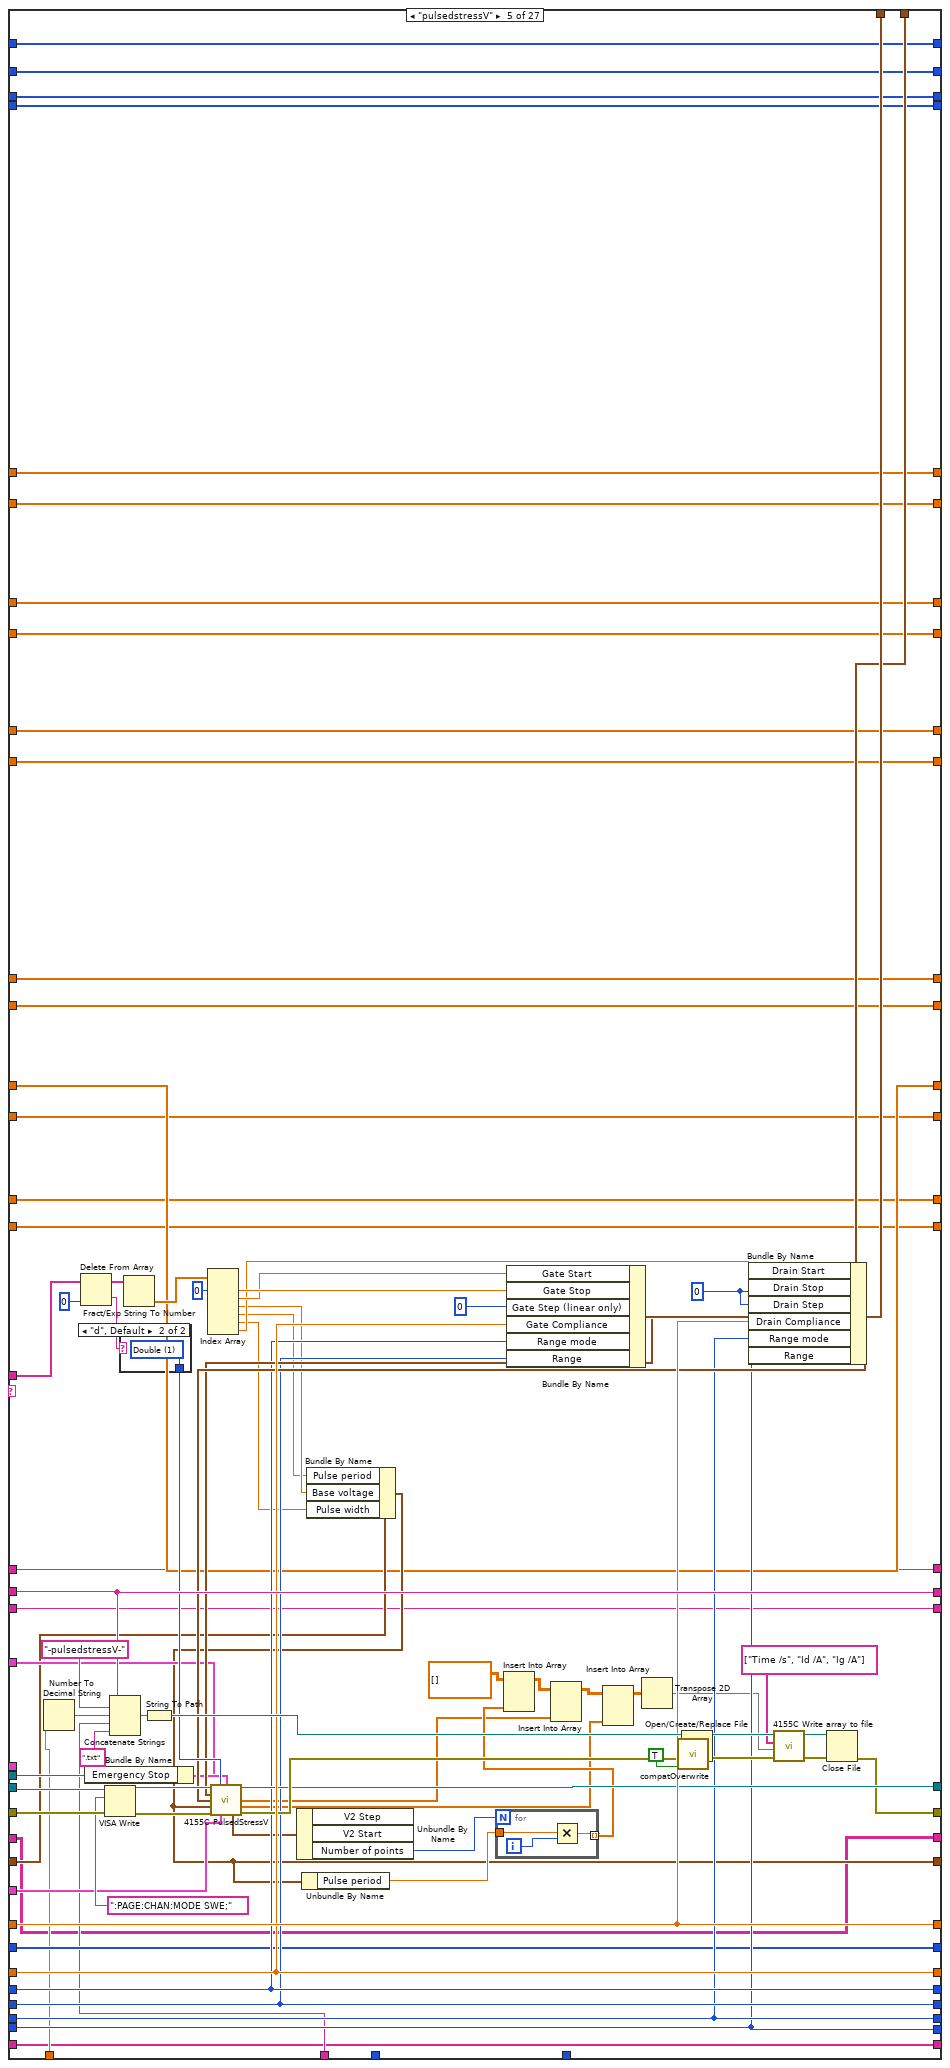
[diagram p13: hidden frame]
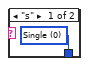
[diagram p14: hidden frame]
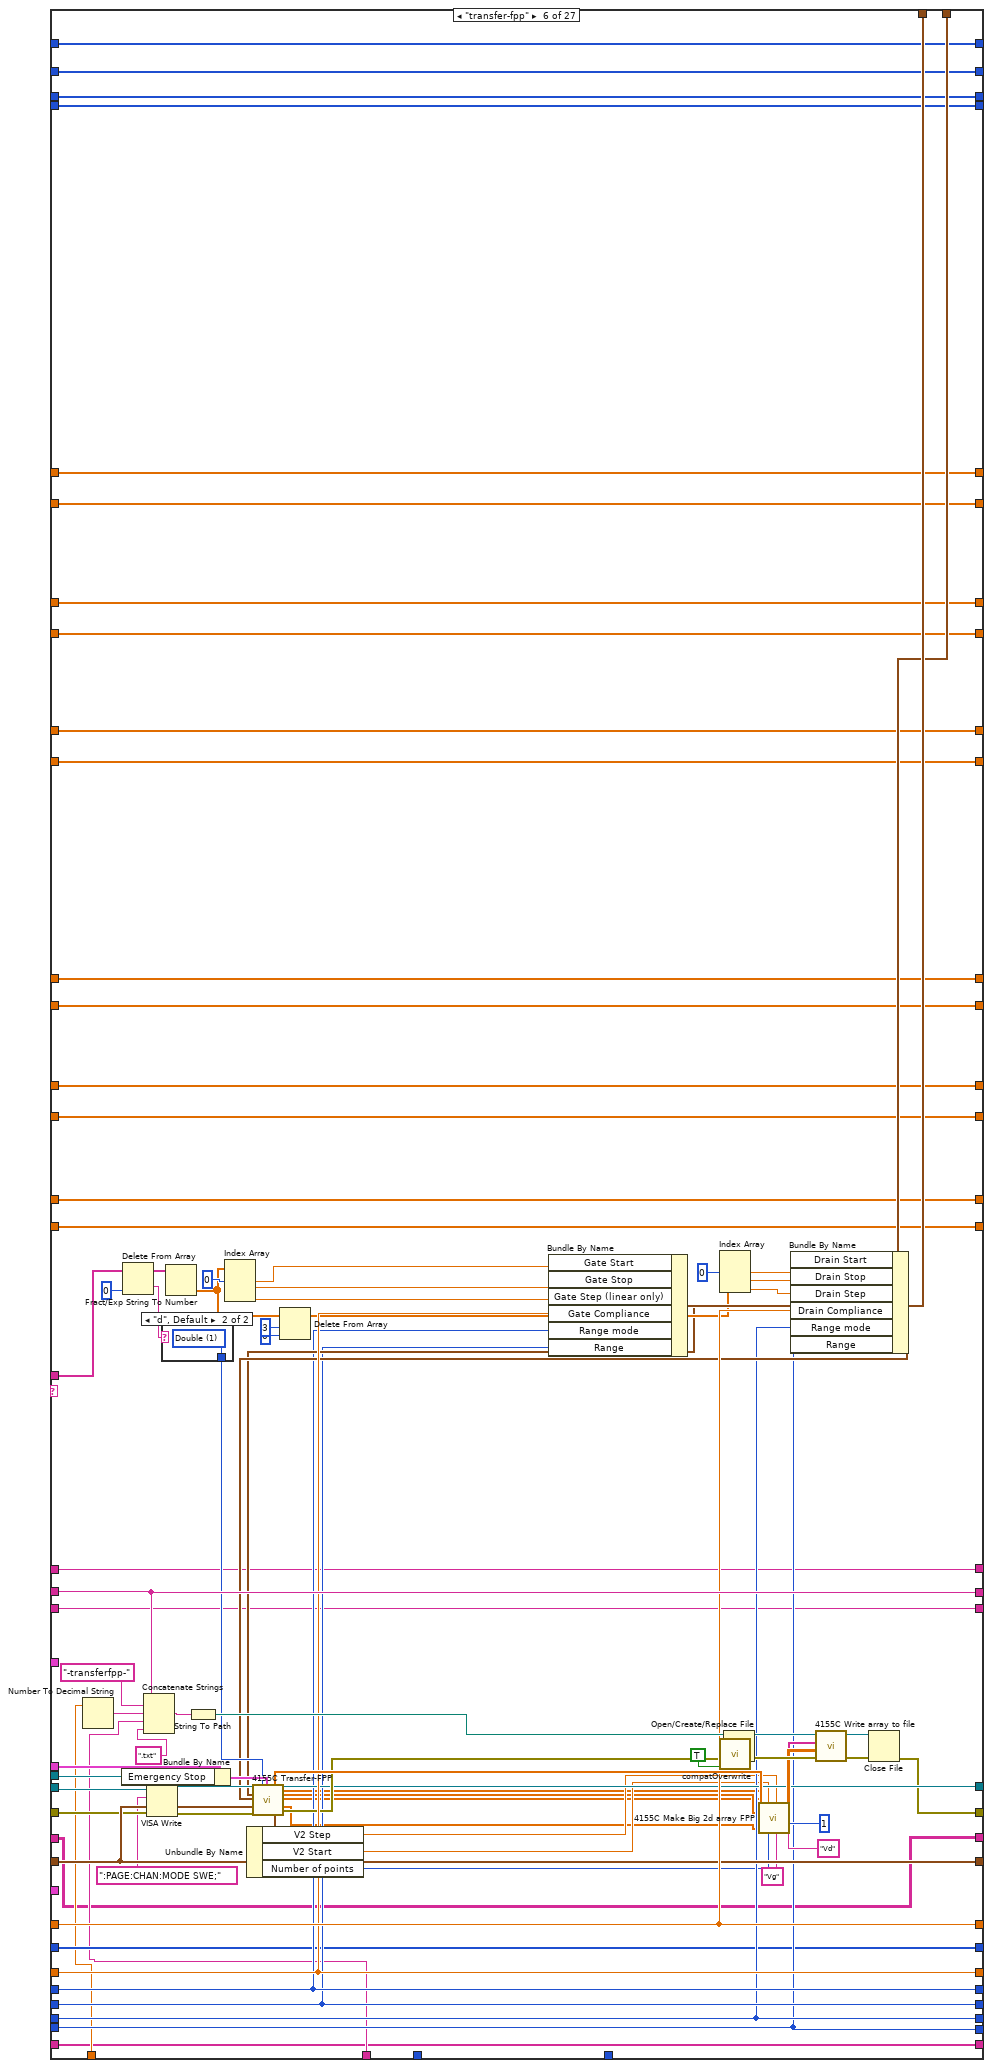
[diagram p15: hidden frame]
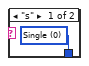
[diagram p16: hidden frame]
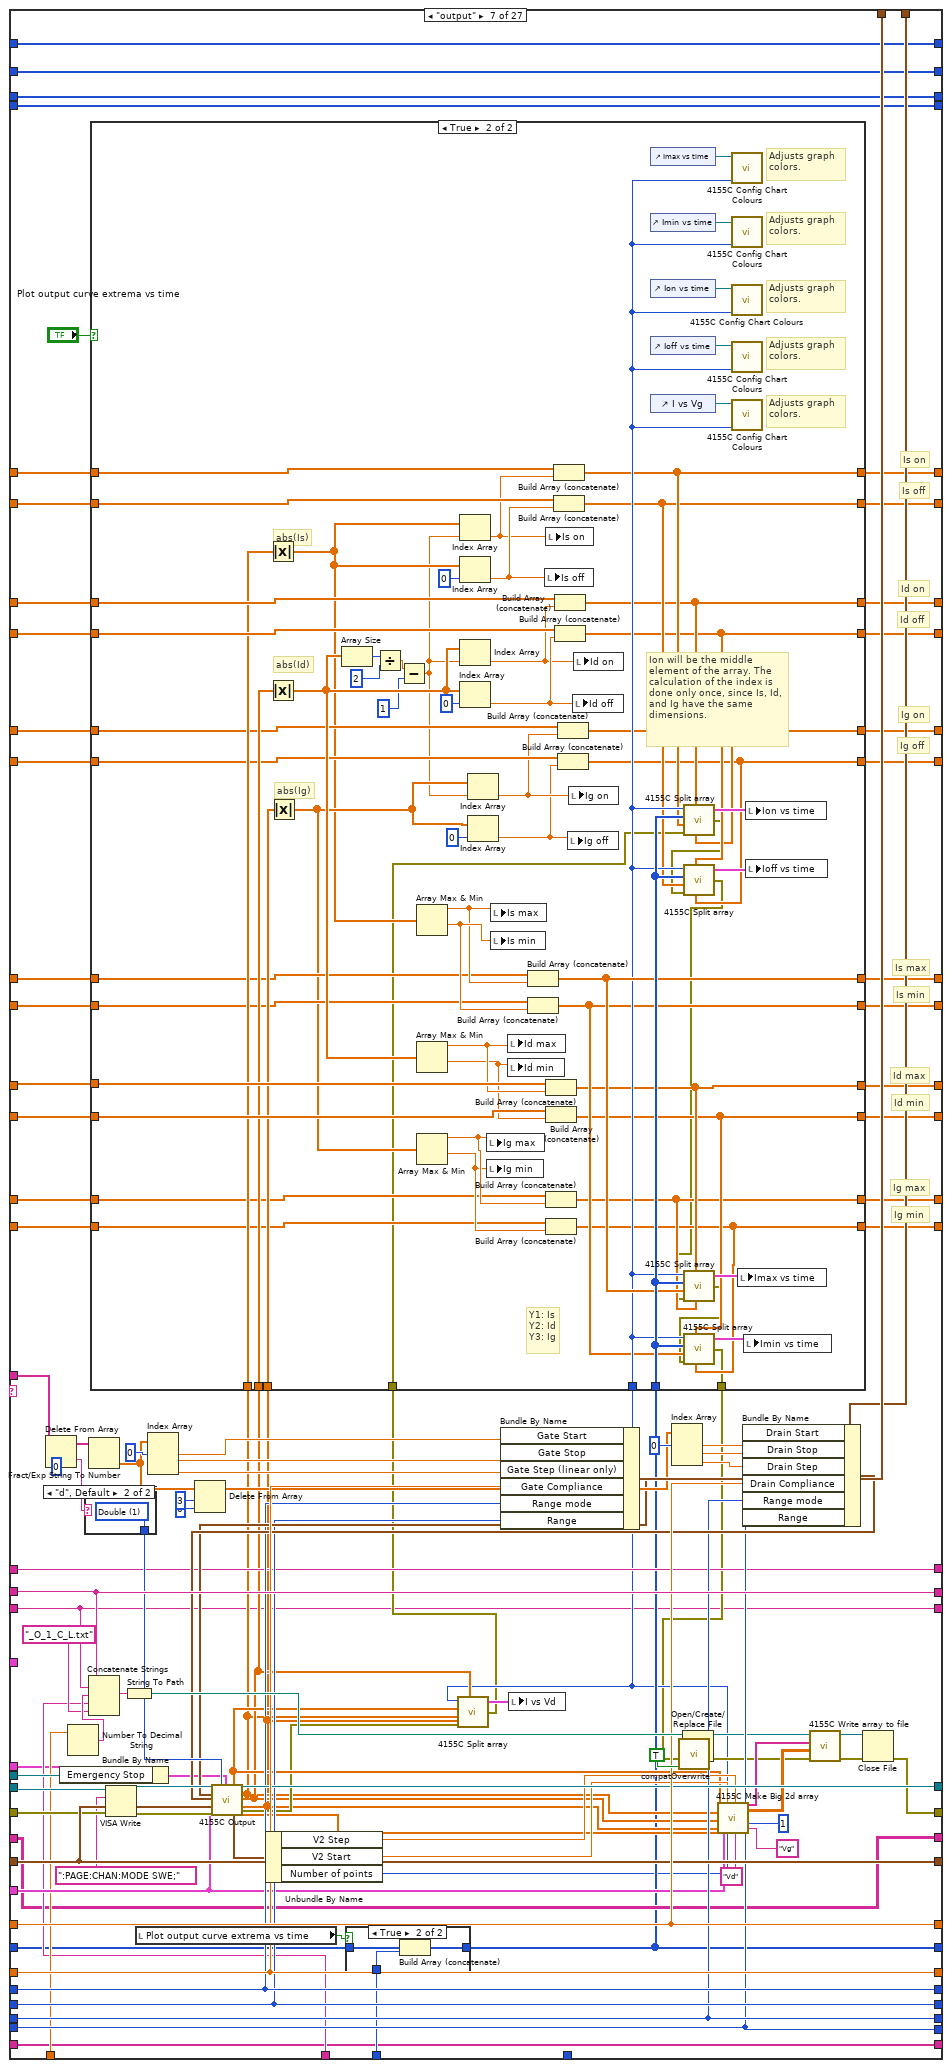
[diagram p17: hidden frame]
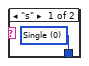
[diagram p20: hidden frame]
diagram:
  w9 = cluster{"Y data in":dbl[], "X data in":dbl[]}[] [] ("I vs Vg")
  w10 = 0.0 ("Is off")
  w11 = 0.0 ("Is on")
  w12 = 0.0 ("Is min")
  w13 = 0.0 ("Is max")
  w62 = u16 1 items=["Reset All", "Partial reset"] ("Type of reset")
  # "Change from previous version:\n\n- Added option for plotting transfer and output curve extrema vs time."
  # "This is a version specific to the SPM pump."
  # "I add 1 to both the \"total lines\" and the \"line running\" indicators because i and N begin from 0, and the script lines begin from 1."
  # "Bugs:\n\n- If using the \"filename\" command, keep in mind that the arrays of the time-dependent data are not re-initialized inbetween filename changes. \n\n- Do not connect the \"error\" wire of a Split block if it has unconnected terminals! It will halt the program."
  # "Array size"
  # "%s option converts a spreadsheet string to an array of strings."
  # "0: No of rows of array\n1: No of cols"
  # "Dimitrios Simatos\nv. 6.4"
  # "Changes from original textcontrol.vi:\n\n- Timestamp appears in filename.\n- (Only) transfer and output curves are plotted.\n- Communication with serial port.\n- Can execute any command, as all pattern matching functions were replaced. Previously, commands with special LabVIEW characters could not be executed.\n- Replaced write to file function with write to text file.\n- Replaced while loop with for loop.\n- Replaced 4155C \"Save File\" function and now the vi can save time-dependent variables.\n- Added clock with start time control and various units.\n- Changed filepath in which the program is saved.\n- Added a serial output log that keeps a history.\n- Tab control.\n- Addition of specialized serial read/write file for the SPM OEM pump.\n- Added halt and hard stop.\n- Added option for plotting transfer and output curve extrema vs time.\n- Corrected bug of \"itime\" command. The command did not allow for settting the integration time value, it allowed to set the category of the integration time (short, medium, long). If the time value was beyond the range of the category, then the SPA used the closest value allowed, whilst staying in the category. So, if the integration time was changed to long, but the integration time value was a short one, then the SPA would measure using the minimum long integration time value and not the value that the user intended."
  # "Search and replace LF with EOL"
  n1 = Equal?(x="integration time", y=u32 0) -> (x = y?=w63:bool)
  n2 = Select(t="Integration time (short)", s=w63, f="Integration time (long)") -> (s? t:f=w14:dbl)
  n3 = call "4155C Get Filename.vi"("error in (no error)"=errorcluster {"status"=FALSE, "code"=0, "source"=""}) -> ("error out"=w57:errorcluster, "path"=w32:path)  [unwired: 2 in, 1 out]
  "Path" <- w32
  n4 = Bundle By Name(cluster="Timings (overwritten by the Front Panel)", "integration time"="integration time", "Short/Long integration time"=w14) -> (w55:T5)
  n5 = Path To String(path=w32) -> (string=w33:string)
  n6 = Search and Replace String(replace all?=TRUE ("replace all? (F)"), input string="Script", search string="\n", replace string="\r\n") -> (result string=w45:string)  [unwired: 4 in, 3 out]
  n7 = Match Pattern(string=w33, regular expression=".txt") -> (before substring=w28:string)  [unwired: 1 in, 3 out]
  n8 = call "4155C Initialise.vi"("VISA resource name in"=refnum<visa-resource-name> "GPIB0::14::INSTR", "Reset"="Full Reset", "Type of reset"=w62, "error in (no error)"=w57, "VISA Timeout Value"=u32 10000) -> ("VISA Resource Name out"=w56:refnum<visa-resource-name>, "error out"=w2:errorcluster)
  n9 = Concatenate Strings(w28, "Suffix (script)") -> (w27:string)
  n10 = Spreadsheet String To Array(delimiter (Tab)="\r\n", format string="%s", spreadsheet string="Script", array type (2D Dbl)="") -> (array=w36:string[][])
  n11 = String To Path(string=w27) -> (path=w5:path)
  n12 = Array Size(array=w36) -> (size(s)=w40:i32[])
  n13 = Initialize Array("") -> (w19:string[])  [unwired: 1 in]
  n14 = Open/Create/Replace File(file path (use dialog)=w5, error in=w2, operation (0:open)=T8."replace or create with confirmation") -> (refnum out=w4:refnum<file>, error out=w3:errorcluster)  [unwired: 3 in, 1 out]
  n15 = Initialize Array(0 ("element")) -> (w21:i32[])  [unwired: 1 in]
  n16 = Initialize Array("") -> (w17:string[][])  [unwired: 2 in]
  n17 = Initialize Array(0.0 ("element")) -> (w23:dbl[])  [unwired: 1 in]
  n18 = Index Array(array=w40, index=0) -> (element=w38:i32)
  n19 = Write to Text File(file (use dialog)=w4, text=w45, error in=w3) -> (error out=w26:errorcluster)  [unwired: 1 in, 2 out]
  n20 = for {
    N: w38 -> [w178]
    tunnel: "SMU4" -> [w214]
    shift-left: "Source/Drain Range" -> [w219]
    shift-right: [w215] -> _
    shift-left: "Source/Drain\nRange mode" -> [w220]
    shift-right: [w216] -> _
    shift-left: "Gate Range" -> [w221]
    shift-right: [w217] -> _
    shift-left: "Gate Range\nmode" -> [w222]
    shift-right: [w218] -> _
    shift-left: "Gate: Compliance" -> [w231]
    shift-right: [w227] -> _
    shift-left: "Drain: Compliance" -> [w232]
    shift-right: [w228] -> _
    shift-left: w55 -> [w233]
    shift-right: [w229] -> w15
    shift-left: w26 -> [w234]
    shift-right: [w124] -> w31
    shift-left: w56 -> [w235]
    shift-right: [w230] -> _
    shift-left: w28 -> [w236]
    shift-right: [w128] -> _
    tunnel: "Panel Controls 2" -> [w213]
    shift-right: [w86] -> _
    shift-left: w23 -> [w212]
    shift-right: [w148] -> _
    shift-left: i32[] [] -> [w208]
    tunnel: w36 -> [w207] mode=indexing
    shift-right: [w85] -> _
    shift-left: w23 -> [w184]
    shift-right: [w118] -> _
    shift-left: w19 -> [w170]
    shift-right: [w149] -> _
    shift-left: w21 -> [w165]
    shift-right: [w130] -> _
    shift-left: w21 -> [w164]
    shift-right: [w163] -> _
    shift-left: "" -> [w162]
    shift-right: [w123] -> _
    shift-left: w21 -> [w145]
    shift-right: [w122] -> _
    shift-left: w21 -> [w129]
    shift-right: [w119] -> _
    shift-left: w17 -> [w121]
    shift-right: [w79] -> _
    shift-left: w23 -> [w107]
    shift-right: [w80] -> _
    shift-left: w23 -> [w106]
    shift-right: [w84] -> _
    shift-left: w23 -> [w95]
    shift-right: [w83] -> _
    shift-left: w23 -> [w94]
    shift-right: [w77] -> _
    shift-left: w23 -> [w93]
    shift-right: [w87] -> _
    shift-left: w23 -> [w92]
    shift-right: [w78] -> _
    shift-left: w23 -> [w91]
    shift-right: [w76] -> _
    shift-left: w23 -> [w90]
    shift-right: [w82] -> _
    shift-left: w23 -> [w89]
    shift-right: [w81] -> _
    shift-left: w23 -> [w88]
    shift-right: [w71] -> _
    shift-left: "Filename (variable part)" -> [w70]
    i -> [w173]
    stop <- "Interrupt program" stop-if-true
    # "Filename prefix"
    # "Is off"
    # "Is on"
    # "Ig off"
    # "Ig on"
    # "Is min"
    # "Is max"
    # "Ig min"
    # "Ig max"
    # "Id min"
    # "Id max"
    # "Id off"
    # "Id on"
    # "Pump status"
    # "Filepath and name"
    # "Pump status"
    # "Limit of command arguments (array columns). Raise if needed."
    # "Serial port data (string)"
    # "Serial port data (table)"
    # "Time array for valve position"
    # "Time array for absolute plunger position"
    # "Valve position"
    # "Absolute plunger position"
    # "Serial port data"
    # "For loop counter"
    # "<-----Equivalent to the 4155C \"Write\" subvi.----->"
    # "Headers"
    # "Save transfer curves in file."
    # "Filepath and name"
    # "Save time-dependent data."
    # "Use the time offset if your measurements do not start at t=0."
    # "Time for Imax, Imin, Ion, Ioff"
    # "Rest of elements of command"
    # "First element of command\n(case select)"
    n21 = Add(x=w173, y=1) -> (x+y=→"Line running":i32)
    n22 = Add(x=w178, y=1) -> (x+y=→"Total lines":i32)
    n23 = Index Array(array=w207, index=0 ("line index")) -> (element=w202:string)
    "Command running:" <- w202
    n24 = control-ref of="Interrupt scan"() -> (w226:refnum<vi>)
    n25 = Spreadsheet String To Array(delimiter (Tab)=" ", format string="%s", spreadsheet string=w202, array type (2D Dbl)=string[] []) -> (array=w200:string[])
    n26 = Delete From Array(array=w200, index=0) -> (deleted portion=w108:string, array with subset deleted=w199:string[])  [unwired: 1 in]
    n27 = call "Elapsed Time"("Reset"="Reset", "Auto Reset"="Auto Reset") -> ("Elapsed Time (s)"=w209:dbl)  [unwired: 10 in, 7 out]
    n28 = case shown="0, Default" "Time Units" {
      tunnel: ["_sec" "_min" "_h"] -> w210
      tunnel: [w240 w244 w247] -> w180
      tunnel: w209 -> [w240 w243 w248]
      frame 0, Default {
      }
      frame 1 {
        n29 = Divide(x=w243, y=60.0) -> (x/y=w244:dbl)
      }
      frame 2 {
        n30 = Divide(x=w248, y=3600.0) -> (x/y=w247:dbl)
      }
    }
    n31 = Add(x=w180, y="Time Offset") -> (x+y=w179:dbl)
    n32 = To Long Integer(number=w179) -> (32bit integer=w146:i32)
    "Elapsed Time" <- w146
    n33 = case shown="\"transfer\"" w108 {
      tunnel: w199 -> [w285 w323 w360 w459 w566 w712 w832 w993 w1020 w1100 w1146 w1190 w1230 w1263 _ _ w1424 w1504 _ w1607 w1670 w1731 w1820 w1901 w1940 w2010 w2064]
      tunnel: w236 -> [w280 w319 w358 w466 w631 w720 w839 w1001 w1043 w1089 w1138 w1183 w1224 w1256 w1294 w1355 w1402 w1486 w1536 w1594 w1657 w1719 w1814 w1897 w1942 w2012 w2066]
      tunnel: w235 -> [w279 w318 w349 w437 w616 w689 w810 w969 w1044 w1090 w1139 w1184 w1225 w1257 w1299 w1357 w1430 w1510 w1540 w1613 w1676 w1737 w1826 w1855 w1946 w2016 w2068]
      tunnel: w234 -> [w278 w317 w348 w436 w615 w688 w809 w966 w1045 w1091 w1140 w1185 w1226 w1258 w1298 w1328 w1429 w1509 w1539 w1612 w1675 w1736 w1825 w1854 w1945 w2015 w2069]
      tunnel: w233 -> [w277 w316 w357 w462 w591 w716 w835 w997 w1053 w1099 w1137 w1182 w1223 w1255 w1297 w1352 w1393 w1478 w1545 w1587 w1650 w1712 w1813 w1896 w1947 w2017 w2071]
      tunnel: w232 -> [w276 w315 w356 w464 w629 w718 w837 w999 w1052 w1098 w1145 w1189 w1229 w1262 w1296 w1337 w1428 w1508 w1548 w1611 w1674 w1735 w1824 w1905 w1948 w2018 w2072]
      tunnel: w231 -> [w275 w314 w355 w463 w628 w717 w836 w998 w1051 w1097 w1144 w1188 w1228 w1261 w1295 w1338 w1403 w1487 w1547 w1595 w1658 w1720 w1815 w1898 w1950 w2019 w2074]
      tunnel: [w279 w318 w347 w461 w626 w714 w834 w995 w1044 w1090 w1139 w1184 w1225 w1257 w1299 w1357 w1394 w1460 w1538 w1588 w1651 w1713 w1766 w1857 w1946 w2016 w2068] -> w230
      tunnel: [w278 w317 w346 w460 w625 w713 w833 w994 w1045 w1091 w1140 w1185 w1226 w1258 w1298 w1327 w1404 w1461 w1537 w1596 w1659 w1721 w1765 w1856 w1944 w2014 w2069] -> w144
      tunnel: [w277 w316 w357 w462 w587 w716 w835 w997 w1046 w1092 w1137 w1182 w1223 w1255 w1297 w1352 w1393 w1478 w1545 w1587 w1650 w1712 w1813 w1896 w1947 w2017 w2071] -> w229
      tunnel: [w276 w315 w356 w464 w629 w718 w837 w999 w1052 w1098 w1145 w1189 w1229 w1262 w1296 w1337 w1428 w1508 w1548 w1611 w1674 w1735 w1824 w1905 w1948 w2018 w2072] -> w228
      tunnel: [w275 w314 w355 w463 w628 w717 w836 w998 w1051 w1097 w1144 w1188 w1228 w1261 w1295 w1338 w1403 w1487 w1547 w1595 w1658 w1720 w1815 w1898 w1950 w2019 w2074] -> w227
      tunnel: [w280 w319 w358 w466 w631 w720 w839 w1001 w1043 w1089 w1138 w1183 w1224 w1256 w1294 w1355 w1402 w1486 w1536 w1594 w1657 w1719 w1814 w1897 w1942 w2012 w2066] -> w128
      tunnel: w226 -> [_ _ _ w468 w635 w725 w841 w1005 _ _ _ _ _ _ _ _ w1399 w1483 _ w1593 w1656 w1718 w1786 w1873 _ _ _]
      tunnel: "Gate" -> [_ _ _ w446 w619 w699 w819 w980 _ _ _ _ _ _ _ _ _ _ _ _ _ _ _ _ _ _ _]
      tunnel: "Drain 2" -> [_ _ _ w445 w618 w698 w818 w979 _ _ _ _ _ _ _ _ _ _ _ _ _ _ _ _ _ _ _]
      tunnel: "Panel Controls" -> [_ _ _ _ _ w697 w738 w978 _ _ _ _ _ _ _ _ _ _ _ _ _ _ _ _ _ _ _]
      tunnel: w222 -> [w274 w313 w354 w430 w609 w682 w803 w964 w1050 w1096 _ w1181 w1222 w1254 w1293 w1339 w1389 w1474 w1541 w1583 w1646 w1708 w1809 w1892 w1951 w2020 w2075]
      tunnel: w221 -> [w273 w312 w353 w429 w608 w681 w802 w963 w1049 w1095 w1143 _ w1213 w1260 w1292 w1340 w1390 w1475 w1542 w1584 w1647 w1709 w1810 w1893 w1952 w2021 w2076]
      tunnel: w220 -> [w272 w311 w352 w428 w607 w680 w801 w962 w1048 w1094 w1142 w1187 w1227 _ w1291 w1341 w1391 w1476 w1543 w1585 w1648 w1710 w1811 w1894 w1953 w2022 w2077]
      tunnel: w219 -> [w271 w310 w351 w427 w606 w679 w800 w965 w1047 w1093 w1141 w1186 _ w1259 w1290 w1342 w1392 w1477 w1544 w1586 w1649 w1711 w1812 w1895 w1954 w2023 w2078]
      tunnel: [w274 w313 w354 w430 w609 w682 w803 w964 w1050 w1096 w1136 w1181 w1222 w1254 w1293 w1339 w1389 w1474 w1541 w1583 w1646 w1708 w1809 w1892 w1951 w2020 w2075] -> w218
      tunnel: [w273 w312 w353 w429 w608 w681 w802 w963 w1049 w1095 w1143 w1173 w1213 w1260 w1292 w1340 w1390 w1475 w1542 w1584 w1647 w1709 w1810 w1893 w1952 w2021 w2076] -> w217
      tunnel: [w272 w311 w352 w428 w607 w680 w801 w962 w1048 w1094 w1142 w1187 w1227 w1253 w1291 w1341 w1391 w1476 w1543 w1585 w1648 w1710 w1811 w1894 w1953 w2022 w2077] -> w216
      tunnel: [w271 w310 w351 w427 w606 w679 w800 w965 w1047 w1093 w1141 w1186 w1214 w1259 w1290 w1342 w1392 w1477 w1544 w1586 w1649 w1711 w1812 w1895 w1954 w2023 w2078] -> w215
      tunnel: w214 -> [_ _ _ w422 w603 _ w795 _ _ _ _ _ _ _ _ _ _ _ _ _ _ _ _ _ _ _ _]
      tunnel: w213 -> [_ _ _ w420 w602 _ _ _ _ _ _ _ _ _ _ _ _ _ _ _ _ _ _ _ _ _ _]
      tunnel: [w270 w306 w344 w377 w579 w669 w751 w951 w1042 w1087 w1135 w1172 w1212 w1252 w1289 w1323 w1381 w1439 w1535 w1572 w1639 w1702 w1763 w1850 w1943 w2013 w2083] -> w86
      tunnel: w212 -> [w270 w306 w344 w417 w579 w669 w791 w951 w1042 w1087 w1135 w1172 w1212 w1252 w1289 w1323 w1381 w1439 w1535 w1572 w1639 w1702 w1763 w1850 w1943 w2013 w2083]
      tunnel: w179 -> [_ _ _ w416 w576 w667 w790 w948 _ _ _ _ _ _ _ w1321 w1379 w1456 _ w1569 w1636 w1699 w1760 w1846 _ _ _]
      tunnel: w210 -> [_ _ _ w413 w575 w665 w787 w947 _ _ _ _ _ _ _ w1319 w1377 w1455 _ w1568 w1635 w1698 w1759 w1847 _ w1981 _]
      tunnel: w146 -> [_ _ _ w409 _ _ w783 _ _ _ _ _ _ _ _ _ _ _ _ _ _ _ _ _ _ w1984 _]
      tunnel: [w269 w305 w343 w381 w578 w668 w755 w950 w1041 w1086 w1134 w1171 w1211 w1251 w1288 w1322 w1380 w1458 w1534 w1571 w1638 w1701 w1762 w1849 w1949 w1993 w2073] -> w148
      tunnel: w208 -> [w269 w305 w343 w412 w578 w668 w786 w950 w1041 w1086 w1134 w1171 w1211 w1251 w1288 w1322 w1380 w1458 w1534 w1571 w1638 w1701 w1762 w1849 w1949 w1993 w2073]
      tunnel: [w268 w304 w342 w376 w574 w664 w750 w946 w1040 w1085 w1133 w1170 w1210 w1250 w1287 w1318 w1376 w1438 w1533 w1567 w1634 w1697 w1758 w1845 w1938 w2009 w2082] -> w85
      tunnel: w184 -> [w268 w304 w342 w408 w574 w664 w782 w946 w1040 w1085 w1133 w1170 w1210 w1250 w1287 w1318 w1376 w1438 w1533 w1567 w1634 w1697 w1758 w1845 w1938 w2009 w2082]
      tunnel: [w267 w303 w341 w401 w573 w663 w775 w945 w1039 w1084 w1132 w1169 w1209 w1249 w1286 w1317 w1375 w1454 w1532 w1566 w1633 w1696 w1757 w1844 w1937 w2008 w2079] -> w118
      tunnel: w170 -> [w267 w303 w341 w401 w573 w663 w775 w945 w1039 w1084 w1132 w1169 w1209 w1249 w1286 w1317 w1375 w1454 w1532 w1566 w1633 w1696 w1757 w1844 w1936 w1982 w2079]
      tunnel: [w266 w302 w340 w400 w572 w662 w774 w944 w1038 w1083 w1131 w1168 w1208 w1248 w1285 w1316 w1374 w1453 w1531 w1565 w1632 w1695 w1756 w1843 w1922 w1995 w2093] -> w149
      tunnel: w165 -> [w266 w302 w340 w400 w572 w662 w774 w944 w1038 w1083 w1131 w1168 w1208 w1248 w1285 w1316 w1374 w1453 w1531 w1565 w1632 w1695 w1756 w1843 w1922 w1994 w2093]
      tunnel: [w265 w301 w339 w399 w571 w661 w773 w943 w1037 w1082 w1130 w1167 w1207 w1247 w1284 w1315 w1373 w1452 w1530 w1564 w1631 w1694 w1755 w1842 w1921 w1977 w2095] -> w130
      tunnel: w164 -> [w265 w301 w339 w399 w571 w661 w773 w943 w1037 w1082 w1130 w1167 w1207 w1247 w1284 w1315 w1373 w1452 w1530 w1564 w1631 w1694 w1755 w1842 w1921 w1975 w2095]
      tunnel: [w264 w300 w338 w398 w570 w660 w772 w942 w1036 w1081 w1129 w1166 w1206 w1246 w1283 w1314 w1372 w1451 w1529 w1563 w1630 w1693 w1754 w1841 w1920 w1974 w2067] -> w163
      tunnel: w162 -> [w264 w300 w338 w398 w570 w660 w772 w942 w1036 w1081 w1129 w1166 w1206 w1246 w1283 w1314 w1372 w1451 w1529 w1563 w1630 w1693 w1754 w1841 w1920 w1985 w2067]
      tunnel: w146 -> [_ _ _ _ _ _ _ _ _ _ _ _ _ _ _ _ _ _ _ _ _ _ _ _ _ w1973 _]
      tunnel: w145 -> [w263 w299 w337 w397 w569 w659 w771 w941 w1035 w1080 w1128 w1165 w1205 w1245 w1282 w1313 w1371 w1450 w1528 w1562 w1629 w1692 w1753 w1840 w1919 w1972 w2094]
      tunnel: [w263 w299 w337 w397 w569 w659 w771 w941 w1035 w1080 w1128 w1165 w1205 w1245 w1282 w1313 w1371 w1450 w1528 w1562 w1629 w1692 w1753 w1840 w1919 w1971 w2094] -> w123
      tunnel: [w262 w298 w336 w396 w568 w658 w770 w940 w1034 w1079 w1127 w1164 w1204 w1244 w1281 w1312 w1370 w1449 w1527 w1561 w1628 w1691 w1752 w1839 w1918 w1970 w2092] -> w122
      tunnel: w129 -> [w262 w298 w336 w396 w568 w658 w770 w940 w1034 w1079 w1127 w1164 w1204 w1244 w1281 w1312 w1370 w1449 w1527 w1561 w1628 w1691 w1752 w1839 w1918 w1969 w2092]
      tunnel: [w261 w297 w335 w395 w567 w657 w769 w939 w1033 w1078 w1126 w1163 w1203 w1243 w1280 w1311 w1369 w1448 w1526 w1560 w1627 w1690 w1751 w1838 w1917 w1967 w2070] -> w119
      tunnel: w121 -> [w261 w297 w335 w395 w567 w657 w769 w939 w1033 w1078 w1126 w1163 w1203 w1243 w1280 w1311 w1369 w1448 w1526 w1560 w1627 w1690 w1751 w1838 w1917 w1966 w2070]
      tunnel: [w259 w295 w333 w370 w564 w655 w744 w937 w1031 w1077 w1125 w1161 w1201 w1241 w1278 w1309 w1368 w1447 w1525 w1559 w1626 w1688 w1750 w1837 w1916 w1965 w2088] -> w79
      tunnel: w107 -> [w259 w295 w333 w394 w564 w655 w768 w937 w1031 w1077 w1125 w1161 w1201 w1241 w1278 w1309 w1368 w1447 w1525 w1559 w1626 w1688 w1750 w1837 w1916 w1965 w2088]
      tunnel: [w260 w296 w334 w371 w565 w656 w745 w938 w1032 w1076 w1124 w1162 w1202 w1242 w1279 w1310 w1367 w1446 w1524 w1558 w1625 w1689 w1749 w1836 w1915 w1964 w2089] -> w80
      tunnel: w106 -> [w260 w296 w334 w393 w565 w656 w767 w938 w1032 w1076 w1124 w1162 w1202 w1242 w1279 w1310 w1367 w1446 w1524 w1558 w1625 w1689 w1749 w1836 w1915 w1964 w2089]
      tunnel: [w252 w288 w326 w375 w561 w653 w749 w935 w1024 w1074 w1122 w1159 w1199 w1239 w1276 w1302 w1360 w1437 w1523 w1551 w1618 w1681 w1742 w1831 w1908 w1963 w2081] -> w84
      tunnel: w95 -> [w252 w288 w326 w389 w561 w653 w763 w935 w1024 w1074 w1122 w1159 w1199 w1239 w1276 w1302 w1360 w1437 w1523 w1551 w1618 w1681 w1742 w1831 w1908 w1963 w2081]
      tunnel: [w251 w287 w325 w374 w562 w654 w748 w936 w1023 w1075 w1123 w1160 w1200 w1240 w1277 w1301 w1359 w1436 w1522 w1550 w1617 w1680 w1741 w1830 w1907 w1962 w2080] -> w83
      tunnel: w94 -> [w251 w287 w325 w388 w562 w654 w762 w936 w1023 w1075 w1123 w1160 w1200 w1240 w1277 w1301 w1359 w1436 w1522 w1550 w1617 w1680 w1741 w1830 w1907 w1962 w2080]
      tunnel: [w254 w290 w328 w380 w560 w651 w754 w933 w1029 w1072 w1120 w1157 w1197 w1237 w1274 w1304 w1362 w1441 w1517 w1553 w1620 w1683 w1744 w1829 w1912 w1960 w2085] -> w77
      tunnel: w93 -> [w254 w290 w328 w387 w560 w651 w761 w933 w1029 w1072 w1120 w1157 w1197 w1237 w1274 w1304 w1362 w1441 w1517 w1553 w1620 w1683 w1744 w1829 w1912 w1960 w2085]
      tunnel: [w253 w289 w327 w378 w563 w652 w752 w934 w1030 w1073 w1121 w1158 w1198 w1238 w1275 w1303 w1361 w1440 w1516 w1552 w1619 w1682 w1743 w1828 w1911 w1961 w2084] -> w87
      tunnel: w92 -> [w253 w289 w327 w386 w563 w652 w760 w934 w1030 w1073 w1121 w1158 w1198 w1238 w1275 w1303 w1361 w1440 w1516 w1552 w1619 w1682 w1743 w1828 w1911 w1961 w2084]
      tunnel: [w256 w292 w330 w369 w559 w649 w743 w931 w1027 w1070 w1118 w1155 w1195 w1235 w1272 w1306 w1364 w1443 w1519 w1555 w1622 w1685 w1746 w1833 w1914 w1958 w2087] -> w78
      tunnel: w91 -> [w256 w292 w330 w385 w559 w649 w759 w931 w1027 w1070 w1118 w1155 w1195 w1235 w1272 w1306 w1364 w1443 w1519 w1555 w1622 w1685 w1746 w1833 w1914 w1958 w2087]
      tunnel: [w255 w291 w329 w368 w558 w650 w742 w932 w1028 w1071 w1119 w1156 w1196 w1236 w1273 w1305 w1363 w1442 w1518 w1554 w1621 w1684 w1745 w1832 w1913 w1959 w2086] -> w76
      tunnel: w90 -> [w255 w291 w329 w384 w558 w650 w758 w932 w1028 w1071 w1119 w1156 w1196 w1236 w1273 w1305 w1363 w1442 w1518 w1554 w1621 w1684 w1745 w1832 w1913 w1959 w2086]
      tunnel: [w258 w294 w332 w373 w557 w647 w747 w929 w1025 w1068 w1116 w1153 w1193 w1233 w1270 w1308 w1366 w1445 w1521 w1557 w1624 w1687 w1748 w1835 w1910 w1956 w2091] -> w82
      tunnel: w89 -> [w258 w294 w332 w383 w557 w647 w757 w929 w1025 w1068 w1116 w1153 w1193 w1233 w1270 w1308 w1366 w1445 w1521 w1557 w1624 w1687 w1748 w1835 w1910 w1956 w2091]
      tunnel: [w257 w293 w331 w372 w556 w648 w746 w930 w1026 w1069 w1117 w1154 w1194 w1234 w1271 w1307 w1365 w1444 w1520 w1556 w1623 w1686 w1747 w1834 w1909 w1957 w2090] -> w81
      tunnel: w88 -> [w257 w293 w331 w382 w556 w648 w756 w930 w1026 w1069 w1117 w1154 w1194 w1234 w1271 w1307 w1365 w1444 w1520 w1556 w1623 w1686 w1747 w1834 w1909 w1957 w2090]
      tunnel: w70 -> [w250 w286 w324 w365 w555 w646 w739 w928 w1022 w1067 w1115 w1152 w1192 w1232 w1269 w1300 w1358 w1435 w1515 w1549 w1616 w1679 w1740 w1827 w1906 w1955 _]
      tunnel: [w250 w286 w324 w365 w555 w646 w739 w928 w1022 w1067 w1115 w1152 w1192 w1232 w1269 w1300 w1358 w1435 w1515 w1549 w1616 w1679 w1740 w1827 w1906 w1955 w2063] -> w71
      frame "wait" {
        n34 = Index Array(array=w285, index=0 ("Index")) -> (element=w283:string)
        n35 = Decimal String To Number(string=w283, default (0L)=u32 0) -> (number=w282:u32)  [unwired: 1 in, 1 out]
        n36 = Wait (ms)(milliseconds to wait=w282) -> ()  [unwired: 1 out]
      }
      frame "wait-min" {
        n37 = Index Array(array=w323, index=0 ("Index")) -> (element=w321:string)
        n38 = Decimal String To Number(string=w321, default (0L)=u32 0) -> (number=w309:u32)  [unwired: 1 in, 1 out]
        n39 = Multiply(x=w309, y=u32 60000) -> (x*y=w308:u32)
        n40 = Wait (ms)(milliseconds to wait=w308) -> ()  [unwired: 1 out]
      }
      frame "standby" {
        n41 = Index Array(array=w360, index=0 ("Index")) -> (element=w350:string)
        n42 = case shown="\"off\", Default" w350 {
          tunnel: [":PAGE:SCON:STAN 0" ":PAGE:SCON:STAN 1"] -> w345
          frame "off", Default {
          }
          frame "on" {
          }
        }
        n43 = VISA Write(VISA resource name=w349, write buffer=w345, error in (no error)=w348) -> (VISA resource name out=w347:refnum<visa-resource-name>, error out=w346:errorcluster)  [unwired: 1 out]
      }
      frame "transfer" {
        # "Is off"
        # "Is on"
        # "Ig off"
        # "Ig on"
        # "Is min"
        # "Is max"
        # "Ig min"
        # "Ig max"
        # "Id min"
        # "Id max"
        # "Id off"
        # "Id on"
        n44 = Delete From Array(array=w459, index=0 ("Index")) -> (deleted portion=w457:string, array with subset deleted=w456:string[])  [unwired: 1 in]
        n45 = Bundle By Name(cluster=w420, "Emergency Stop"=w468) -> (w421:T2)
        n46 = Number To Decimal String(number=w416) -> (decimal integer string=w415:string)  [unwired: 1 in]
        n47 = case shown="\"d\", Default" w457 {
          tunnel: [w553 w554] -> w455
          frame "s" {
            w553 = u16 0 items=["Single", "Double"] ("sweep mode")
          }
          frame "d", Default {
            w554 = u16 1 items=["Single", "Double"] ("sweep mode")
          }
        }
        n48 = Fract/Exp String To Number(string=w456) -> (number=w441:dbl[])  [unwired: 3 in, 1 out]
        n49 = Concatenate Strings(w466, w365, w415, w413, "_T_1_C_L.txt" ("Suffix (transfer)")) -> (w467:string)
        n50 = VISA Write(VISA resource name=w437, write buffer=":PAGE:CHAN:MODE SWE;" ("write buffer (\"\")"), error in (no error)=w436) -> (VISA resource name out=w434:refnum<visa-resource-name>, error out=w435:errorcluster)  [unwired: 1 out]
        n51 = local read "Plot transfer curve extrema vs time"() -> (w363:bool)
        n52 = String To Path(string=w467) -> (path=w465:path)
        n53 = Index Array(array=w441, index #1=0 ("Index")) -> (element #1=w454:dbl, element #2=w453:dbl, element #3=w452:dbl)  [unwired: 2 in]
        n54 = Delete From Array(array=w441, length=3 ("Length"), index=0 ("Index")) -> (array with subset deleted=w439:dbl[])  [unwired: 1 out]
        n55 = case shown="True" w363 {
          tunnel: w412 -> [w470 w473]
          tunnel: w409 -> [_ w472]
          tunnel: [w470 w471] -> w381
          frame False {
          }
          frame True {
            n56 = Build Array (concatenate)(w473, w472) -> (w471:i32[])
          }
        }
        n57 = Bundle By Name(cluster=w446, "Gate Start"=w454, "Gate Stop"=w453, "Gate Step (linear only)"=w452, "Gate Compliance"=w463, "Range mode"=w430, "Range"=w429) -> (w431:T6)
        n58 = Index Array(array=w439, index #1=0 ("Index")) -> (element #1=w449:dbl, element #2=w448:dbl, element #3=w447:dbl)  [unwired: 2 in]
        n59 = call <vilib>:"compatOverwrite.vi"("overwrite (F)"=TRUE) -> ("overwrite?"=w419:T8)
        n60 = Bundle By Name(cluster=w445, "Drain Start"=w449, "Drain Stop"=w448, "Drain Step"=w447, "Drain Compliance"=w464, "Range mode"=w428, "Range"=w427) -> (w432:T7)
        n61 = call "4155C Transfer.vi"("VISA resource name in"=w434, "Gate"=w431, "Drain"=w432, "Timings"=w462, "error in (no error)"=w435, "SMU4"=w422, "sweep mode"=w455, "Panel Controls"=w421) -> ("VG"=w418:dbl[], "Outparams"=w426:T9, "VISA Resource Name out"=w461:refnum<visa-resource-name>, "IS"=w391:dbl[], "ID"=w392:dbl[], "IG"=w390:dbl[], "error out"=w410:errorcluster, "SMU4"=w423:dbl[])  [unwired: 12 in]
        n62 = Unbundle By Name(w426) -> ("V2 Step"=w425:dbl, "V2 Start"=w424:dbl, "Number of points"=w379:i32)
        n63 = call "4155C Split array.vi"("Number of VAR2 steps"=w379, "Y2 data in"=w392, "X data in"=w418, "Y1 data in"=w391, "Y3 data in"=w390, "error in (no error)"=w410) -> ("Array of clusters"=w411:cluster{"Y data in":dbl[], "X data in":dbl[]}[], "error out"=w367:errorcluster)  [unwired: 1 in]
        n64 = case shown="True" "Plot transfer curve extrema vs time" {
          tunnel: w417 -> [w482 w552]
          tunnel: w408 -> [w483 w547]
          tunnel: w394 -> [w476 w543]
          tunnel: w393 -> [w477 w542]
          tunnel: w392 -> [_ w539]
          tunnel: w391 -> [_ w537]
          tunnel: w390 -> [_ w536]
          tunnel: w389 -> [w484 w532]
          tunnel: w388 -> [w485 w531]
          tunnel: w387 -> [w480 w528]
          tunnel: w386 -> [w481 w527]
          tunnel: w385 -> [w475 w524]
          tunnel: w384 -> [w474 w523]
          tunnel: w383 -> [w479 w520]
          tunnel: w382 -> [w478 w519]
          tunnel: w381 -> [_ w512]
          tunnel: [w480 w507] -> w380
          tunnel: w379 -> [_ w506]
          tunnel: [w481 w505] -> w378
          tunnel: [w482 w504] -> w377
          tunnel: [w483 w503] -> w376
          tunnel: [w484 w502] -> w375
          tunnel: [w485 w501] -> w374
          tunnel: [w479 w500] -> w373
          tunnel: [w478 w499] -> w372
          tunnel: [w477 w498] -> w371
          tunnel: [w476 w497] -> w370
          tunnel: [w475 w496] -> w369
          tunnel: [w474 w495] -> w368
          tunnel: w367 -> [w486 w494]
          tunnel: [w486 w490] -> w366
          frame False {
          }
          frame True {
            # "Adjusts graph colors."
            # "Adjusts graph colors."
            # "Ion will be the middle element of the array. The calculation of the index is done only once, since Is, Id, and Ig have the same dimensions."
            # "abs(Ig)"
            # "abs(Is)"
            # "Y1: Is\nY2: Id\nY3: Ig"
            # "abs(Id)"
            # "Adjusts graph colors."
            # "Adjusts graph colors."
            # "Adjusts graph colors."
            n65 = Absolute Value(x=w537) -> (abs(x)=w522:dbl[])
            n66 = Absolute Value(x=w539) -> (abs(x)=w538:dbl[])
            n67 = Absolute Value(x=w536) -> (abs(x)=w525:dbl[])
            n68 = Array Size(array=w538) -> (size(s)=w546:i32)
            n69 = Divide(x=w546, y=2) -> (x/y=w489:dbl)
            n70 = Subtract(x=w489, y=1) -> (x-y=w488:dbl)
            n71 = Array Max & Min(array=w522) -> (max value=w529:dbl, min value=w530:dbl)  [unwired: 2 out]
            n72 = Array Max & Min(array=w538) -> (max value=w551:dbl, min value=w535:dbl)  [unwired: 2 out]
            n73 = Array Max & Min(array=w525) -> (max value=w534:dbl, min value=w533:dbl)  [unwired: 2 out]
            n74 = Index Array(array=w522, index=w488) -> (element=w513:dbl)
            n75 = Index Array(array=w522, index=0) -> (element=w514:dbl)
            n76 = Index Array(array=w538, index=w488) -> (element=w515:dbl)
            n77 = Index Array(array=w538, index=0) -> (element=w516:dbl)
            n78 = Index Array(array=w525, index=w488) -> (element=w518:dbl)
            n79 = Index Array(array=w525, index=0) -> (element=w517:dbl)
            n80 = local write "Ig max"(w534) -> ()
            n81 = local write "Ig min"(w533) -> ()
            n82 = local write "Is max"(w529) -> ()
            n83 = local write "Is min"(w530) -> ()
            n84 = local write "Id max"(w551) -> ()
            n85 = local write "Id min"(w535) -> ()
            n86 = Build Array (concatenate)(w528, w529) -> (w507:dbl[])
            n87 = Build Array (concatenate)(w527, w530) -> (w505:dbl[])
            n88 = local write "Is off"(w514) -> ()
            n89 = local write "Is on"(w513) -> ()
            n90 = Build Array (concatenate)(w552, w551) -> (w504:dbl[])
            n91 = Build Array (concatenate)(w547, w535) -> (w503:dbl[])
            n92 = Build Array (concatenate)(w532, w534) -> (w502:dbl[])
            n93 = Build Array (concatenate)(w531, w533) -> (w501:dbl[])
            n94 = Build Array (concatenate)(w520, w513) -> (w500:dbl[])
            n95 = Build Array (concatenate)(w519, w514) -> (w499:dbl[])
            n96 = Build Array (concatenate)(w542, w515) -> (w498:dbl[])
            n97 = Build Array (concatenate)(w543, w516) -> (w497:dbl[])
            n98 = Build Array (concatenate)(w524, w518) -> (w496:dbl[])
            n99 = Build Array (concatenate)(w523, w517) -> (w495:dbl[])
            n100 = local write "Ig off"(w517) -> ()
            n101 = local write "Ig on"(w518) -> ()
            n102 = local write "Id off"(w516) -> ()
            n103 = local write "Id on"(w515) -> ()
            n104 = control-ref of="Imax vs time"() -> (w541:refnum<vi>)
            n105 = control-ref of="Imin vs time"() -> (w540:refnum<vi>)
            n106 = control-ref of="Ion vs time"() -> (w509:refnum<vi>)
            n107 = control-ref of="Ioff vs time"() -> (w508:refnum<vi>)
            n108 = control-ref of="I vs Vg"() -> (w550:refnum<vi>)
            n109 = call "4155C Split array.vi"("Number of VAR2 steps"=w506, "Y2 data in"=w498, "X data in"=w512, "Y1 data in"=w500, "Y3 data in"=w496, "error in (no error)"=w494) -> ("Array of clusters"=w510:cluster{"Y data in":dbl[], "X data in":dbl[]}[], "error out"=w493:errorcluster)  [unwired: 1 in]
            n110 = call "4155C Split array.vi"("Number of VAR2 steps"=w506, "Y2 data in"=w497, "X data in"=w512, "Y1 data in"=w499, "Y3 data in"=w495, "error in (no error)"=w493) -> ("Array of clusters"=w511:cluster{"Y data in":dbl[], "X data in":dbl[]}[], "error out"=w492:errorcluster)  [unwired: 1 in]
            n111 = call "4155C Split array.vi"("Number of VAR2 steps"=w506, "Y2 data in"=w504, "X data in"=w512, "Y1 data in"=w507, "Y3 data in"=w502, "error in (no error)"=w492) -> ("Array of clusters"=w549:cluster{"Y data in":dbl[], "X data in":dbl[]}[], "error out"=w491:errorcluster)  [unwired: 1 in]
            n112 = call "4155C Split array.vi"("Number of VAR2 steps"=w506, "Y2 data in"=w503, "X data in"=w512, "Y1 data in"=w505, "Y3 data in"=w501, "error in (no error)"=w491) -> ("Array of clusters"=w548:cluster{"Y data in":dbl[], "X data in":dbl[]}[], "error out"=w490:errorcluster)  [unwired: 1 in]
            n113 = call "4155C Config Chart Colours.vi"("Numeric"=w506, "XY Graph 2"=w541) -> ()  [unwired: 6 in]
            n114 = call "4155C Config Chart Colours.vi"("Numeric"=w506, "XY Graph 2"=w540) -> ()  [unwired: 6 in]
            n115 = call "4155C Config Chart Colours.vi"("Numeric"=w506, "XY Graph 2"=w509) -> ()  [unwired: 6 in]
            n116 = call "4155C Config Chart Colours.vi"("Numeric"=w506, "XY Graph 2"=w508) -> ()  [unwired: 6 in]
            n117 = call "4155C Config Chart Colours.vi"("Numeric"=w506, "XY Graph 2"=w550) -> ()  [unwired: 6 in]
            n118 = local write "Imax vs time"(w549) -> ()
            n119 = local write "Imin vs time"(w548) -> ()
            n120 = local write "Ion vs time"(w510) -> ()
            n121 = local write "Ioff vs time"(w511) -> ()
          }
        }
        n122 = local write "I vs Vg"(w411) -> ()
        n123 = Open/Create/Replace File(file path (use dialog)=w465, error in=w366, operation (0:open)=w419) -> (refnum out=w406:refnum<file>, error out=w404:errorcluster)  [unwired: 3 in, 1 out]
        n124 = call "4155C Make Big 2d array.vi"("1D Var1"=w418, "1d IS"=w391, "1d ID"=w392, "1d IG"=w390, "1d SMU4"=w423, "SMU4"=w422, "VAR2 START"=w424, "Number of VAR2 steps"=w379, "VAR2 STEP"=w425, "VAR1 Name"="Vg", "Decimal places in header"=i8 1, "VAR2 Name"="Vd") -> ("Header array"=w407:string[], "Data array"=w405:dbl[][])  [unwired: 14 in]
        n125 = call "4155C Write array to file.vi"("Byte Stream File Refnum"=w406, "Header"=w407, "Data Array"=w405, "error in (no error)"=w404) -> ("dup refnum"=w403:refnum<file>, "error out"=w402:errorcluster)  [unwired: 1 in]
        n126 = Close File(refnum=w403, error in=w402) -> (error out=w460:errorcluster)  [unwired: 1 out]
      }
      frame "pulsedstressV" {
        w585 = 0
        n127 = Number To Decimal String(number=w576) -> (decimal integer string=w632:string)  [unwired: 1 in]
        n128 = Delete From Array(array=w566, index=0 ("Index")) -> (deleted portion=w623:string, array with subset deleted=w622:string[])  [unwired: 1 in]
        n129 = Bundle By Name(cluster=w602, "Emergency Stop"=w635) -> (w604:T2)
        n130 = VISA Write(VISA resource name=w616, write buffer=":PAGE:CHAN:MODE SWE;" ("write buffer (\"\")"), error in (no error)=w615) -> (VISA resource name out=w613:refnum<visa-resource-name>, error out=w614:errorcluster)  [unwired: 1 out]
        n131 = Concatenate Strings(w631, "-pulsedstressV-" ("Substring"), w632, w575, ".txt" ("Substring")) -> (w634:string)
        n132 = case shown="\"d\", Default" w623 {
          tunnel: [w644 w645] -> w621
          frame "s" {
            w644 = u16 0 items=["Single", "Double"] ("sweep mode")
          }
          frame "d", Default {
            w645 = u16 1 items=["Single", "Double"] ("sweep mode")
          }
        }
        n133 = Fract/Exp String To Number(string=w622) -> (number=w617:dbl[])  [unwired: 3 in, 1 out]
        n134 = String To Path(string=w634) -> (path=w630:path)
        n135 = Index Array(array=w617, index #1=0 ("Index")) -> (element #1=w594:dbl, element #2=w593:dbl, element #3=w590:dbl, element #4=w589:dbl, element #5=w588:dbl, element #6=w592:dbl)  [unwired: 5 in]
        n136 = Bundle By Name(cluster=w591, "Pulse period"=w589, "Base voltage"=w590, "Pulse width"=w588) -> (w587:T5)
        n137 = Unbundle By Name(w587) -> ("Pulse period"=w595:dbl)
        n138 = Bundle By Name(cluster=w619, "Gate Start"=w593, "Gate Stop"=w594, "Gate Step (linear only)"=0, "Gate Compliance"=w628, "Range mode"=w609, "Range"=w608) -> (w610:T6)
        n139 = call <vilib>:"compatOverwrite.vi"("overwrite (F)"=TRUE) -> ("overwrite?"=w580:T8)
        n140 = Bundle By Name(cluster=w618, "Drain Start"=w592, "Drain Stop"=w585, "Drain Step"=w585, "Drain Compliance"=w629, "Range mode"=w607, "Range"=w606) -> (w611:T7)
        n141 = call "4155C PulsedStressV.vi"("VISA resource name in"=w613, "sweep mode"=w621, "Panel Controls"=w604, "Gate"=w610, "Drain"=w611, "Timings"=w587, "error in (no error)"=w614, "SMU4"=w603) -> ("VISA Resource Name out"=w626:refnum<visa-resource-name>, "ID"=w583:dbl[], "IG"=w581:dbl[], "Outparams"=w605:T9, "error out"=w627:errorcluster)  [unwired: 3 in]
        n142 = Unbundle By Name(w605) -> ("Number of points"=w582:i32)  [unwired: 2 out]
        n143 = for {
          N: w582 -> [_]
          tunnel: [w641] -> w584 mode=indexing
          tunnel: w595 -> [w643]
          i -> [w642]
          n144 = Multiply(x=w643, y=w642) -> (x*y=w641:dbl)
        }
        n145 = Insert Into Array(array=dbl[][] [] ("Input Array"), new element=w584) -> (w596:dbl[][])  [unwired: 2 in]
        n146 = Insert Into Array(array=w596, new element=w583) -> (w601:dbl[][])  [unwired: 2 in]
        n147 = Insert Into Array(array=w601, new element=w581) -> (w600:dbl[][])  [unwired: 2 in]
        n148 = Transpose 2D Array(2D array=w600) -> (transposed array=w599:dbl[][])
        n149 = Open/Create/Replace File(file path (use dialog)=w630, error in=w627, operation (0:open)=w580) -> (refnum out=w638:refnum<file>, error out=w639:errorcluster)  [unwired: 3 in, 1 out]
        n150 = call "4155C Write array to file.vi"("Byte Stream File Refnum"=w638, "Header"=string[] ["Time /s", "Id /A", "Ig /A"], "Data Array"=w599, "error in (no error)"=w639) -> ("dup refnum"=w636:refnum<file>, "error out"=w637:errorcluster)  [unwired: 1 in]
        n151 = Close File(refnum=w636, error in=w637) -> (error out=w625:errorcluster)  [unwired: 1 out]
      }
      frame "transfer-fpp" {
        n152 = Number To Decimal String(number=w667) -> (decimal integer string=w721:string)  [unwired: 1 in]
        n153 = Bundle By Name(cluster=w697, "Emergency Stop"=w725) -> (w733:T1)
        n154 = Delete From Array(array=w712, index=0 ("Index")) -> (deleted portion=w710:string, array with subset deleted=w709:string[])  [unwired: 1 in]
        n155 = Concatenate Strings(w720, "-transferfpp-" ("Substring"), w721, w665, ".txt" ("Substring")) -> (w723:string)
        n156 = VISA Write(VISA resource name=w689, write buffer=":PAGE:CHAN:MODE SWE;" ("write buffer (\"\")"), error in (no error)=w688) -> (VISA resource name out=w686:refnum<visa-resource-name>, error out=w687:errorcluster)  [unwired: 1 out]
        n157 = case shown="\"d\", Default" w710 {
          tunnel: [w734 w735] -> w708
          frame "s" {
            w734 = u16 0 items=["Single", "Double"] ("sweep mode")
          }
          frame "d", Default {
            w735 = u16 1 items=["Single", "Double"] ("sweep mode")
          }
        }
        n158 = Fract/Exp String To Number(string=w709) -> (number=w693:dbl[])  [unwired: 3 in, 1 out]
        n159 = String To Path(string=w723) -> (path=w719:path)
        n160 = Index Array(array=w693, index #1=0 ("Index")) -> (element #1=w707:dbl, element #2=w706:dbl, element #3=w705:dbl)  [unwired: 2 in]
        n161 = Delete From Array(array=w693, length=3 ("Length"), index=0 ("Index")) -> (array with subset deleted=w691:dbl[])  [unwired: 1 out]
        n162 = Bundle By Name(cluster=w699, "Gate Start"=w707, "Gate Stop"=w706, "Gate Step (linear only)"=w705, "Gate Compliance"=w717, "Range mode"=w682, "Range"=w681) -> (w683:T6)
        n163 = Index Array(array=w691, index #1=0 ("Index")) -> (element #1=w702:dbl, element #2=w701:dbl, element #3=w700:dbl)  [unwired: 2 in]
        n164 = call <vilib>:"compatOverwrite.vi"("overwrite (F)"=TRUE) -> ("overwrite?"=w670:T8)
        n165 = Bundle By Name(cluster=w698, "Drain Start"=w702, "Drain Stop"=w701, "Drain Step"=w700, "Drain Compliance"=w718, "Range mode"=w680, "Range"=w679) -> (w684:T7)
        n166 = call "4155C Transfer-FPP.vi"("VISA resource name in"=w686, "Gate"=w683, "Drain"=w684, "Timings"=w716, "error in (no error)"=w687, "sweep mode"=w708, "Panel Controls"=w733) -> ("VG"=w724:dbl[], "Outparams"=w678:T9, "VISA Resource Name out"=w714:refnum<visa-resource-name>, "Vprobe2"=w674:dbl[], "ID"=w673:dbl[], "IG"=w672:dbl[], "Vprobe1"=w671:dbl[], "error out"=w715:errorcluster)  [unwired: 13 in]
        n167 = Unbundle By Name(w678) -> ("V2 Step"=w677:dbl, "V2 Start"=w676:dbl, "Number of points"=w675:i32)
        n168 = Open/Create/Replace File(file path (use dialog)=w719, error in=w715, operation (0:open)=w670) -> (refnum out=w730:refnum<file>, error out=w731:errorcluster)  [unwired: 3 in, 1 out]
        n169 = call "4155C Make Big 2d array FPP.vi"("1D Var1"=w724, "1d ID"=w673, "1d Vp2"=w674, "1d IG"=w672, "1d Vp1"=w671, "VAR2 START"=w676, "Number of VAR2 steps"=w675, "VAR2 STEP"=w677, "VAR1 Name"="Vg", "Decimal places in header"=i8 1, "VAR2 Name"="Vd") -> ("Header array"=w726:string[], "Data array"=w727:dbl[][])  [unwired: 15 in]
        n170 = call "4155C Write array to file.vi"("Byte Stream File Refnum"=w730, "Header"=w726, "Data Array"=w727, "error in (no error)"=w731) -> ("dup refnum"=w728:refnum<file>, "error out"=w729:errorcluster)  [unwired: 1 in]
        n171 = Close File(refnum=w728, error in=w729) -> (error out=w713:errorcluster)  [unwired: 1 out]
      }
      frame "output" {
        # "Is off"
        # "Is on"
        # "Ig off"
        # "Ig on"
        # "Is min"
        # "Is max"
        # "Ig min"
        # "Ig max"
        # "Id min"
        # "Id max"
        # "Id off"
        # "Id on"
        n172 = Delete From Array(array=w832, index=0 ("Index")) -> (deleted portion=w830:string, array with subset deleted=w829:string[])  [unwired: 1 in]
        n173 = Bundle By Name(cluster=w738, "Emergency Stop"=w841) -> (w794:T1)
        n174 = Number To Decimal String(number=w790) -> (decimal integer string=w789:string)  [unwired: 1 in]
        n175 = case shown="\"d\", Default" w830 {
          tunnel: [w926 w927] -> w828
          frame "s" {
            w926 = u16 0 items=["Single", "Double"] ("sweep mode")
          }
          frame "d", Default {
            w927 = u16 1 items=["Single", "Double"] ("sweep mode")
          }
        }
        n176 = Fract/Exp String To Number(string=w829) -> (number=w814:dbl[])  [unwired: 3 in, 1 out]
        n177 = Concatenate Strings(w839, w739, w789, w787, "_O_1_C_L.txt" ("Suffix (transfer)")) -> (w840:string)
        n178 = VISA Write(VISA resource name=w810, write buffer=":PAGE:CHAN:MODE SWE;" ("write buffer (\"\")"), error in (no error)=w809) -> (VISA resource name out=w807:refnum<visa-resource-name>, error out=w808:errorcluster)  [unwired: 1 out]
        n179 = String To Path(string=w840) -> (path=w838:path)
        n180 = local read "Plot output curve extrema vs time"() -> (w736:bool)
        n181 = Index Array(array=w814, index #1=0 ("Index")) -> (element #1=w827:dbl, element #2=w826:dbl, element #3=w825:dbl)  [unwired: 2 in]
        n182 = Delete From Array(array=w814, length=3 ("Length"), index=0 ("Index")) -> (array with subset deleted=w812:dbl[])  [unwired: 1 out]
        n183 = case shown="True" w736 {
          tunnel: w786 -> [w843 w846]
          tunnel: w783 -> [_ w845]
          tunnel: [w843 w844] -> w755
          frame False {
          }
          frame True {
            n184 = Build Array (concatenate)(w846, w845) -> (w844:i32[])
          }
        }
        n185 = Bundle By Name(cluster=w819, "Gate Start"=w827, "Gate Stop"=w826, "Gate Step (linear only)"=w825, "Gate Compliance"=w836, "Range mode"=w803, "Range"=w802) -> (w804:T6)
        n186 = Index Array(array=w812, index #1=0 ("Index")) -> (element #1=w822:dbl, element #2=w821:dbl, element #3=w820:dbl)  [unwired: 2 in]
        n187 = call <vilib>:"compatOverwrite.vi"("overwrite (F)"=TRUE) -> ("overwrite?"=w793:T8)
        n188 = Bundle By Name(cluster=w818, "Drain Start"=w822, "Drain Stop"=w821, "Drain Step"=w820, "Drain Compliance"=w837, "Range mode"=w801, "Range"=w800) -> (w805:T7)
        n189 = call "4155C Output.vi"("VISA resource name in"=w807, "Gate"=w804, "Drain"=w805, "Timings"=w835, "error in (no error)"=w808, "SMU4"=w795, "sweep mode"=w828, "Panel controls"=w794) -> ("VD"=w792:dbl[], "Outparams"=w799:T9, "VISA Resource Name out"=w834:refnum<visa-resource-name>, "IS"=w765:dbl[], "ID"=w766:dbl[], "IG"=w764:dbl[], "error out"=w784:errorcluster, "SMU4"=w796:dbl[])  [unwired: 12 in]
        n190 = Unbundle By Name(w799) -> ("V2 Step"=w798:dbl, "V2 Start"=w797:dbl, "Number of points"=w753:i32)
        n191 = call "4155C Split array.vi"("Number of VAR2 steps"=w753, "Y2 data in"=w766, "X data in"=w792, "Y1 data in"=w765, "Y3 data in"=w764, "error in (no error)"=w784) -> ("Array of clusters"=w785:cluster{"Y data in":dbl[], "X data in":dbl[]}[], "error out"=w741:errorcluster)  [unwired: 1 in]
        n192 = case shown="True" "Plot output curve extrema vs time" {
          tunnel: w791 -> [w850 w925]
          tunnel: w782 -> [w849 w920]
          tunnel: w768 -> [w855 w916]
          tunnel: w767 -> [w856 w915]
          tunnel: w766 -> [_ w912]
          tunnel: w765 -> [_ w910]
          tunnel: w764 -> [_ w909]
          tunnel: w763 -> [w848 w905]
          tunnel: w762 -> [w847 w904]
          tunnel: w761 -> [w852 w901]
          tunnel: w760 -> [w851 w900]
          tunnel: w759 -> [w854 w897]
          tunnel: w758 -> [w853 w896]
          tunnel: w757 -> [w858 w893]
          tunnel: w756 -> [w857 w892]
          tunnel: w755 -> [_ w885]
          tunnel: [w852 w880] -> w754
          tunnel: w753 -> [_ w879]
          tunnel: [w851 w878] -> w752
          tunnel: [w850 w877] -> w751
          tunnel: [w849 w876] -> w750
          tunnel: [w848 w875] -> w749
          tunnel: [w847 w874] -> w748
          tunnel: [w858 w873] -> w747
          tunnel: [w857 w872] -> w746
          tunnel: [w856 w871] -> w745
          tunnel: [w855 w870] -> w744
          tunnel: [w854 w869] -> w743
          tunnel: [w853 w868] -> w742
          tunnel: w741 -> [w859 w867]
          tunnel: [w859 w863] -> w740
          frame False {
          }
          frame True {
            # "Adjusts graph colors."
            # "Adjusts graph colors."
            # "Ion will be the middle element of the array. The calculation of the index is done only once, since Is, Id, and Ig have the same dimensions."
            # "abs(Ig)"
            # "abs(Is)"
            # "Y1: Is\nY2: Id\nY3: Ig"
            # "abs(Id)"
            # "Adjusts graph colors."
            # "Adjusts graph colors."
            # "Adjusts graph colors."
            n193 = Absolute Value(x=w910) -> (abs(x)=w895:dbl[])
            n194 = Absolute Value(x=w912) -> (abs(x)=w911:dbl[])
            n195 = Absolute Value(x=w909) -> (abs(x)=w898:dbl[])
            n196 = Array Size(array=w911) -> (size(s)=w919:i32)
            n197 = Divide(x=w919, y=2) -> (x/y=w862:dbl)
            n198 = Subtract(x=w862, y=1) -> (x-y=w861:dbl)
            n199 = Array Max & Min(array=w895) -> (max value=w902:dbl, min value=w903:dbl)  [unwired: 2 out]
            n200 = Array Max & Min(array=w911) -> (max value=w924:dbl, min value=w908:dbl)  [unwired: 2 out]
            n201 = Array Max & Min(array=w898) -> (max value=w907:dbl, min value=w906:dbl)  [unwired: 2 out]
            n202 = Index Array(array=w895, index=w861) -> (element=w886:dbl)
            n203 = Index Array(array=w895, index=0) -> (element=w887:dbl)
            n204 = Index Array(array=w911, index=w861) -> (element=w888:dbl)
            n205 = Index Array(array=w911, index=0) -> (element=w889:dbl)
            n206 = Index Array(array=w898, index=w861) -> (element=w891:dbl)
            n207 = Index Array(array=w898, index=0) -> (element=w890:dbl)
            n208 = local write "Ig max"(w907) -> ()
            n209 = local write "Ig min"(w906) -> ()
            n210 = local write "Is max"(w902) -> ()
            n211 = local write "Is min"(w903) -> ()
            n212 = local write "Id max"(w924) -> ()
            n213 = local write "Id min"(w908) -> ()
            n214 = Build Array (concatenate)(w901, w902) -> (w880:dbl[])
            n215 = Build Array (concatenate)(w900, w903) -> (w878:dbl[])
            n216 = local write "Is off"(w887) -> ()
            n217 = local write "Is on"(w886) -> ()
            n218 = Build Array (concatenate)(w925, w924) -> (w877:dbl[])
            n219 = Build Array (concatenate)(w920, w908) -> (w876:dbl[])
            n220 = Build Array (concatenate)(w905, w907) -> (w875:dbl[])
            n221 = Build Array (concatenate)(w904, w906) -> (w874:dbl[])
            n222 = Build Array (concatenate)(w893, w886) -> (w873:dbl[])
            n223 = Build Array (concatenate)(w892, w887) -> (w872:dbl[])
            n224 = Build Array (concatenate)(w915, w888) -> (w871:dbl[])
            n225 = Build Array (concatenate)(w916, w889) -> (w870:dbl[])
            n226 = Build Array (concatenate)(w897, w891) -> (w869:dbl[])
            n227 = Build Array (concatenate)(w896, w890) -> (w868:dbl[])
            n228 = local write "Ig off"(w890) -> ()
            n229 = local write "Ig on"(w891) -> ()
            n230 = local write "Id off"(w889) -> ()
            n231 = local write "Id on"(w888) -> ()
            n232 = control-ref of="Imax vs time"() -> (w914:refnum<vi>)
            n233 = control-ref of="Imin vs time"() -> (w913:refnum<vi>)
            n234 = control-ref of="Ion vs time"() -> (w882:refnum<vi>)
            n235 = control-ref of="Ioff vs time"() -> (w881:refnum<vi>)
            n236 = control-ref of="I vs Vg"() -> (w923:refnum<vi>)
            n237 = call "4155C Split array.vi"("Number of VAR2 steps"=w879, "Y2 data in"=w871, "X data in"=w885, "Y1 data in"=w873, "Y3 data in"=w869, "error in (no error)"=w867) -> ("Array of clusters"=w883:cluster{"Y data in":dbl[], "X data in":dbl[]}[], "error out"=w866:errorcluster)  [unwired: 1 in]
            n238 = call "4155C Split array.vi"("Number of VAR2 steps"=w879, "Y2 data in"=w870, "X data in"=w885, "Y1 data in"=w872, "Y3 data in"=w868, "error in (no error)"=w866) -> ("Array of clusters"=w884:cluster{"Y data in":dbl[], "X data in":dbl[]}[], "error out"=w865:errorcluster)  [unwired: 1 in]
            n239 = call "4155C Split array.vi"("Number of VAR2 steps"=w879, "Y2 data in"=w877, "X data in"=w885, "Y1 data in"=w880, "Y3 data in"=w875, "error in (no error)"=w865) -> ("Array of clusters"=w922:cluster{"Y data in":dbl[], "X data in":dbl[]}[], "error out"=w864:errorcluster)  [unwired: 1 in]
            n240 = call "4155C Split array.vi"("Number of VAR2 steps"=w879, "Y2 data in"=w876, "X data in"=w885, "Y1 data in"=w878, "Y3 data in"=w874, "error in (no error)"=w864) -> ("Array of clusters"=w921:cluster{"Y data in":dbl[], "X data in":dbl[]}[], "error out"=w863:errorcluster)  [unwired: 1 in]
            n241 = call "4155C Config Chart Colours.vi"("Numeric"=w879, "XY Graph 2"=w914) -> ()  [unwired: 6 in]
            n242 = call "4155C Config Chart Colours.vi"("Numeric"=w879, "XY Graph 2"=w913) -> ()  [unwired: 6 in]
            n243 = call "4155C Config Chart Colours.vi"("Numeric"=w879, "XY Graph 2"=w882) -> ()  [unwired: 6 in]
            n244 = call "4155C Config Chart Colours.vi"("Numeric"=w879, "XY Graph 2"=w881) -> ()  [unwired: 6 in]
            n245 = call "4155C Config Chart Colours.vi"("Numeric"=w879, "XY Graph 2"=w923) -> ()  [unwired: 6 in]
            n246 = local write "Imax vs time"(w922) -> ()
            n247 = local write "Imin vs time"(w921) -> ()
            n248 = local write "Ion vs time"(w883) -> ()
            n249 = local write "Ioff vs time"(w884) -> ()
          }
        }
        n250 = local write "I vs Vd"(w785) -> ()
        n251 = Open/Create/Replace File(file path (use dialog)=w838, error in=w740, operation (0:open)=w793) -> (refnum out=w780:refnum<file>, error out=w778:errorcluster)  [unwired: 3 in, 1 out]
        n252 = call "4155C Make Big 2d array.vi"("1D Var1"=w792, "1d IS"=w765, "1d ID"=w766, "1d IG"=w764, "1d SMU4"=w796, "SMU4"=w795, "VAR2 START"=w797, "Number of VAR2 steps"=w753, "VAR2 STEP"=w798, "VAR1 Name"="Vd", "Decimal places in header"=i8 1, "VAR2 Name"="Vg") -> ("Header array"=w781:string[], "Data array"=w779:dbl[][])  [unwired: 14 in]
        n253 = call "4155C Write array to file.vi"("Byte Stream File Refnum"=w780, "Header"=w781, "Data Array"=w779, "error in (no error)"=w778) -> ("dup refnum"=w777:refnum<file>, "error out"=w776:errorcluster)  [unwired: 1 in]
        n254 = Close File(refnum=w777, error in=w776) -> (error out=w833:errorcluster)  [unwired: 1 out]
      }
      frame "output-fpp" {
        n255 = Number To Decimal String(number=w948) -> (decimal integer string=w1002:string)  [unwired: 1 in]
        n256 = Bundle By Name(cluster=w978, "Emergency Stop"=w1005) -> (w1015:T1)
        n257 = Delete From Array(array=w993, index=0 ("Index")) -> (deleted portion=w991:string, array with subset deleted=w990:string[])  [unwired: 1 in]
        n258 = VISA Write(VISA resource name=w969, write buffer=":PAGE:CHAN:MODE SWE;" ("write buffer (\"\")"), error in (no error)=w966) -> (VISA resource name out=w968:refnum<visa-resource-name>, error out=w967:errorcluster)  [unwired: 1 out]
        n259 = Concatenate Strings(w1001, "-outputfpp-" ("Substring"), w1002, w947, ".txt" ("Substring")) -> (w1004:string)
        n260 = case shown="\"d\", Default" w991 {
          tunnel: [w1016 w1017] -> w989
          frame "s" {
            w1016 = u16 0 items=["Single", "Double"] ("sweep mode")
          }
          frame "d", Default {
            w1017 = u16 1 items=["Single", "Double"] ("sweep mode")
          }
        }
        n261 = Fract/Exp String To Number(string=w990) -> (number=w972:dbl[])  [unwired: 3 in, 1 out]
        n262 = String To Path(string=w1004) -> (path=w1000:path)
        n263 = Index Array(array=w972, index #1=0 ("Index")) -> (element #1=w988:dbl, element #2=w987:dbl, element #3=w986:dbl)  [unwired: 2 in]
        n264 = Delete From Array(array=w972, length=3 ("Length"), index=0 ("Index")) -> (array with subset deleted=w971:dbl[])  [unwired: 1 out]
        n265 = Bundle By Name(cluster=w980, "Gate Start"=w988, "Gate Stop"=w987, "Gate Step (linear only)"=w986, "Gate Compliance"=w998, "Range mode"=w964, "Range"=w963) -> (w1014:T6)
        n266 = Index Array(array=w971, index #1=0 ("Index")) -> (element #1=w983:dbl, element #2=w982:dbl, element #3=w981:dbl)  [unwired: 2 in]
        n267 = call <vilib>:"compatOverwrite.vi"("overwrite (F)"=TRUE) -> ("overwrite?"=w952:T8)
        n268 = Bundle By Name(cluster=w979, "Drain Start"=w983, "Drain Stop"=w982, "Drain Step"=w981, "Drain Compliance"=w999, "Range mode"=w962, "Range"=w965) -> (w1013:T7)
        n269 = call "4155C Output-FPP.vi"("VISA resource name in"=w968, "Gate"=w1014, "Drain"=w1013, "Timings"=w997, "error in (no error)"=w967, "sweep mode"=w989, "Panel controls"=w1015) -> ("VD"=w957:dbl[], "Outparams"=w960:T9, "VISA Resource Name out"=w995:refnum<visa-resource-name>, "Vprobe2"=w956:dbl[], "ID"=w955:dbl[], "IG"=w954:dbl[], "Vprobe1"=w953:dbl[], "error out"=w996:errorcluster)  [unwired: 13 in]
        n270 = Unbundle By Name(w960) -> ("V2 Step"=w961:dbl, "V2 Start"=w959:dbl, "Number of points"=w958:i32)
        n271 = Open/Create/Replace File(file path (use dialog)=w1000, error in=w996, operation (0:open)=w952) -> (refnum out=w1010:refnum<file>, error out=w1011:errorcluster)  [unwired: 3 in, 1 out]
        n272 = call "4155C Make Big 2d array FPP.vi"("1D Var1"=w957, "1d ID"=w955, "1d Vp2"=w956, "1d IG"=w954, "1d Vp1"=w953, "VAR2 START"=w959, "Number of VAR2 steps"=w958, "VAR2 STEP"=w961, "VAR1 Name"="Vd", "Decimal places in header"=i8 1, "VAR2 Name"="Vg") -> ("Header array"=w1006:string[], "Data array"=w1007:dbl[][])  [unwired: 15 in]
        n273 = call "4155C Write array to file.vi"("Byte Stream File Refnum"=w1010, "Header"=w1006, "Data Array"=w1007, "error in (no error)"=w1011) -> ("dup refnum"=w1008:refnum<file>, "error out"=w1009:errorcluster)  [unwired: 1 in]
        n274 = Close File(refnum=w1008, error in=w1009) -> (error out=w994:errorcluster)  [unwired: 1 out]
      }
      frame "itime" {
        n275 = Delete From Array(array=w1020, index=1) -> (deleted portion=w1019:string)  [unwired: 1 in, 1 out]
        n276 = Delete From Array(array=w1020, index=0 ("Index")) -> (deleted portion=w1054:string)  [unwired: 1 in, 1 out]
        n277 = Fract/Exp String To Number(string=w1019) -> (number=w1018:dbl)  [unwired: 3 in, 1 out]
        n278 = case shown="\"l\"" w1054 {
          tunnel: w1053 -> [w1059 w1061 w1065]
          tunnel: [w1058 w1060 w1064] -> w1046
          tunnel: w1018 -> [w1056 _ w1063]
          frame "s" {
            w1057 = u32 0 items=["short  ", "medium  ", "long  "] ("integration time 2")
            n279 = Bundle By Name(cluster=w1059, "integration time"=w1057, "Short/Long integration time"=w1056) -> (w1058:T5)
          }
          frame "m", Default {
            w1062 = u32 1 items=["short  ", "medium  ", "long  "] ("integration time 2")
            n280 = Bundle By Name(cluster=w1061, "integration time"=w1062) -> (w1060:T5)
          }
          frame "l" {
            w1066 = u32 2 items=["short  ", "medium  ", "long  "] ("integration time 2")
            n281 = Bundle By Name(cluster=w1065, "integration time"=w1066, "Short/Long integration time"=w1063) -> (w1064:T5)
          }
        }
      }
      frame "pulsed" {
        n282 = Delete From Array(array=w1100, index=0 ("Index")) -> (deleted portion=w1101:string, array with subset deleted=w1088:string[])  [unwired: 1 in]
        n283 = case shown="\"on\", Default" w1101 {
          tunnel: w1099 -> [w1111 w1114]
          tunnel: [w1110 w1113] -> w1092
          tunnel: w1088 -> [w1108 _]
          frame "on", Default {
            w1109 = u16 1 items=["Continuous", "Pulsed"] ("sweep method")
            n284 = Fract/Exp String To Number(string=w1108) -> (number=w1106:dbl[])  [unwired: 3 in, 1 out]
            n285 = Index Array(array=w1106, index #1=0 ("Index")) -> (element #1=w1105:dbl, element #2=w1104:dbl, element #3=w1103:dbl)  [unwired: 2 in]
            n286 = Bundle By Name(cluster=w1111, "sweep method"=w1109, "Pulse period"=w1105, "Base voltage"=w1104, "Pulse width"=w1103) -> (w1110:T5)
          }
          frame "off" {
            w1112 = u16 0 items=["Continuous", "Pulsed"] ("sweep method")
            n287 = Bundle By Name(cluster=w1114, "sweep method"=w1112) -> (w1113:T5)
          }
        }
      }
      frame "gaterangemode" {
        n288 = Delete From Array(array=w1146, index=0 ("Index")) -> (deleted portion=w1147:string)  [unwired: 1 in, 1 out]
        n289 = case shown="\"f\"" w1147 {
          tunnel: [w1149 w1150 w1151] -> w1136
          frame "a", Default {
            w1149 = u16 0 items=["Auto", "Limited", "Fixed"] ("Gate Range\nmode 2")
          }
          frame "f" {
            w1150 = u16 2 items=["Auto", "Limited", "Fixed"] ("Gate Range\nmode 2")
          }
          frame "l" {
            w1151 = u16 1 items=["Auto", "Limited", "Fixed"] ("Gate Range\nmode 2")
          }
        }
      }
      frame "gaterange" {
        (unwired) u8 11 items=["10fA  ", "100fA  ", "1nA  ", "10nA", "100nA", "1uA", "10uA", "100uA", "1mA", "10mA", "100mA", "1A"] ("Gate Range 2")
        n290 = Delete From Array(array=w1190, index=0 ("Index")) -> (deleted portion=w1180:string)  [unwired: 1 in, 1 out]
        n291 = Scan Value(string=w1180, format string="") -> (value=w1178:dbl)  [unwired: 1 in, 1 out]
        n292 = Logarithm Base 10(1:w1178) -> (0:w1177:dbl)
        n293 = Round To Nearest(number=w1177) -> (nearest integer value=w1176:dbl)
        n294 = Add(x=w1176, y=11.0) -> (x+y=w1174:dbl)
        n295 = To Unsigned Byte Integer(number=w1174) -> (unsigned 8bit integer=w1173:u8)
      }
      frame "drainrange" {
        (unwired) u8 11 items=["10fA  ", "100fA  ", "1nA  ", "10nA", "100nA", "1uA", "10uA", "100uA", "1mA", "10mA", "100mA", "1A"] ("Gate Range 2")
        n296 = Delete From Array(array=w1230, index=0 ("Index")) -> (deleted portion=w1221:string)  [unwired: 1 in, 1 out]
        n297 = Scan Value(string=w1221, format string="") -> (value=w1219:dbl)  [unwired: 1 in, 1 out]
        n298 = Logarithm Base 10(1:w1219) -> (0:w1218:dbl)
        n299 = Round To Nearest(number=w1218) -> (nearest integer value=w1217:dbl)
        n300 = Add(x=w1217, y=11.0) -> (x+y=w1215:dbl)
        n301 = To Unsigned Byte Integer(number=w1215) -> (unsigned 8bit integer=w1214:u8)
      }
      frame "drainrangemode" {
        n302 = Delete From Array(array=w1263, index=0 ("Index")) -> (deleted portion=w1264:string)  [unwired: 1 in, 1 out]
        n303 = case shown="\"f\"" w1264 {
          tunnel: [w1266 w1267 w1268] -> w1253
          frame "a", Default {
            w1266 = u16 0 items=["Auto", "Limited", "Fixed"] ("Gate Range\nmode 2")
          }
          frame "f" {
            w1267 = u16 2 items=["Auto", "Limited", "Fixed"] ("Gate Range\nmode 2")
          }
          frame "l" {
            w1268 = u16 1 items=["Auto", "Limited", "Fixed"] ("Gate Range\nmode 2")
          }
        }
      }
      frame "Error", Default {
      }
      frame "logfile" {
        n304 = Number To Decimal String(number=w1321) -> (decimal integer string=w1356:string)  [unwired: 1 in]
        n305 = Concatenate Strings(w1355, "logfile" ("Substring"), w1356, w1319, ".txt" ("Substring")) -> (w1353:string)
        n306 = String To Path(string=w1353) -> (path=w1326:path)
        n307 = Unbundle(w1352) -> ("integration time"=w1351:u32, "Short/Long integration time"=w1350:dbl, "hold time (sec)"=w1349:dbl, "delay time (sec)"=w1348:dbl, "Step Time (0 disables)"=w1347:dbl, "sweep method"=w1346:u16, "Pulse period"=w1345:dbl, "Base voltage"=w1344:dbl, "Pulse width"=w1343:dbl)
        n308 = Build Array(w1351, w1350, w1349, w1348, w1347, w1346, w1345, w1344, w1343, w1337, w1338, w1339, w1340, w1341, w1342) -> (w1330:dbl[])
        n309 = Insert Into Array(array=dbl[][] [] ("Input Array"), new element=w1330) -> (w1329:dbl[][])  [unwired: 2 in]
        n310 = call <vilib>:"compatOverwrite.vi"("overwrite (F)"=TRUE) -> ("overwrite?"=w1324:T8)
        n311 = Open/Create/Replace File(file path (use dialog)=w1326, error in=w1328, operation (0:open)=w1324) -> (refnum out=w1334:refnum<file>, error out=w1333:errorcluster)  [unwired: 3 in, 1 out]
        n312 = call "4155C Write array to file.vi"("Byte Stream File Refnum"=w1334, "Header"=string[] ["Int Time", "Short/Long Itime", "Hold time", "Delay time", "Step time", "Sweep method", "Pulse period", "Base Voltage", "Pulse width", "Drain compliance", "Gate compliance", "Gate range mode", "Gate range", "S/D range mode", "S/D range"], "Data Array"=w1329, "error in (no error)"=w1333) -> ("dup refnum"=w1336:refnum<file>, "error out"=w1335:errorcluster)  [unwired: 1 in]
        n313 = Close File(refnum=w1336, error in=w1335) -> (error out=w1327:errorcluster)  [unwired: 1 out]
      }
      frame "sample" {
        n314 = Number To Decimal String(number=w1379) -> (decimal integer string=w1427:string)  [unwired: 1 in]
        n315 = Fract/Exp String To Number(string=w1424) -> (number=w1385:dbl[])  [unwired: 3 in, 1 out]
        n316 = Concatenate Strings(w1402, "-sample-" ("Substring"), w1427, w1377, ".txt" ("Substring")) -> (w1425:string)
        n317 = Index Array(array=w1385, index=0 ("Index")) -> (element=w1422:dbl)
        n318 = String To Path(string=w1425) -> (path=w1406:path)
        n319 = Index Array(array=w1385, index=2 ("Index")) -> (element=w1418:dbl)
        n320 = Index Array(array=w1385, index=3 ("Index")) -> (element=w1387:dbl)
        n321 = Index Array(array=w1385, index=4 ("Index")) -> (element=w1384:dbl)
        n322 = call "4155C Config Sampling Measurements.vi"("Sampling interval"=w1384, "Sample time"=w1387, "Display on/off"=TRUE, "Timings"=w1393, "Num Points"=w1418, "error in (no error)"=w1429, "Drain Compliance"=w1428, "Gate Compliance"=w1403, "VISA session"=w1430) -> ("error out"=w1431:errorcluster, "dup VISA resource name"=w1432:refnum<visa-resource-name>)  [unwired: 1 in]
        n323 = Index Array(array=w1385, index=1 ("Index")) -> (element=w1419:dbl)
        n324 = call "4155C Take Sample.vi"("Emergency Stop"=w1399, "error in (no error)"=w1431, "Vd"=w1419, "Vg"=w1422, "VISA resource name in"=w1432) -> ("error out"=w1397:errorcluster, "Id"=w1434:dbl[], "Ig"=w1408:dbl[], "VISA Resource Name out"=w1395:refnum<visa-resource-name>, "Is"=w1433:dbl[], "Time"=w1412:dbl[])  [unwired: 1 in]
        n325 = Insert Into Array(array=dbl[][] [] ("Input Array"), new element=w1412) -> (w1411:dbl[][])  [unwired: 2 in]
        n326 = Insert Into Array(array=w1411, new element=w1408) -> (w1410:dbl[][])  [unwired: 2 in]
        n327 = Insert Into Array(array=w1410, new element=w1434) -> (w1409:dbl[][])  [unwired: 2 in]
        n328 = VISA Write(VISA resource name=w1395, write buffer=":DISP ON" ("write buffer (\"\")"), error in (no error)=w1397) -> (VISA resource name out=w1394:refnum<visa-resource-name>, error out=w1396:errorcluster)  [unwired: 1 out]
        n329 = Insert Into Array(array=w1409, new element=w1433) -> (w1401:dbl[][])  [unwired: 2 in]
        n330 = Transpose 2D Array(2D array=w1401) -> (transposed array=w1400:dbl[][])
        n331 = call <vilib>:"compatOverwrite.vi"("overwrite (F)"=TRUE) -> ("overwrite?"=w1382:T8)
        n332 = Open/Create/Replace File(file path (use dialog)=w1406, error in=w1396, operation (0:open)=w1382) -> (refnum out=w1415:refnum<file>, error out=w1414:errorcluster)  [unwired: 3 in, 1 out]
        n333 = call "4155C Write array to file.vi"("Byte Stream File Refnum"=w1415, "Header"=string[] ["Time /s", "Ig /A", "Id /A", "Is /A"], "Data Array"=w1400, "error in (no error)"=w1414) -> ("dup refnum"=w1417:refnum<file>, "error out"=w1416:errorcluster)  [unwired: 1 in]
        n334 = Close File(refnum=w1417, error in=w1416) -> (error out=w1404:errorcluster)  [unwired: 1 out]
      }
      frame "samplei" {
        n335 = Number To Decimal String(number=w1456) -> (decimal integer string=w1507:string)  [unwired: 1 in]
        n336 = Concatenate Strings(w1486, "-samplei-" ("Substring"), w1507, w1455, ".txt" ("Substring")) -> (w1505:string)
        n337 = Fract/Exp String To Number(string=w1504) -> (number=w1471:dbl[])  [unwired: 3 in, 1 out]
        n338 = String To Path(string=w1505) -> (path=w1489:path)
        n339 = Index Array(array=w1471, index=4 ("Index")) -> (element=w1465:dbl)
        n340 = Index Array(array=w1471, index=3 ("Index")) -> (element=w1466:dbl)
        n341 = Index Array(array=w1471, index=1 ("Index")) -> (element=w1468:dbl)
        n342 = Index Array(array=w1471, index=0 ("Index")) -> (element=w1469:dbl)
        n343 = Index Array(array=w1471, index=2 ("Index")) -> (element=w1467:dbl)
        n344 = call "4155C Config SamplingI Measurements.vi"("Sample time"=w1467, "Display on/off"=TRUE, "Timings"=w1478, "Num Points"=w1468, "error in (no error)"=w1509, "Sampling interval"=w1466, "VISA session"=w1510) -> ("error out"=w1511:errorcluster, "dup VISA resource name"=w1512:refnum<visa-resource-name>)  [unwired: 3 in]
        n345 = call "4155C Take SampleI.vi"("Emergency Stop"=w1483, "error in (no error)"=w1511, "Idg 2"=w1469, "Vdg compliance 2"=w1465, "VISA resource name in"=w1512) -> ("error out"=w1481:errorcluster, "Idg"=w1514:dbl[], "Vdg"=w1491:dbl[], "VISA Resource Name out"=w1479:refnum<visa-resource-name>, "Is"=w1513:dbl[], "Time"=w1495:dbl[])  [unwired: 1 in]
        n346 = Insert Into Array(array=dbl[][] [] ("Input Array"), new element=w1495) -> (w1494:dbl[][])  [unwired: 2 in]
        n347 = Insert Into Array(array=w1494, new element=w1491) -> (w1493:dbl[][])  [unwired: 2 in]
        n348 = Insert Into Array(array=w1493, new element=w1514) -> (w1492:dbl[][])  [unwired: 2 in]
        n349 = VISA Write(VISA resource name=w1479, write buffer=":DISP ON" ("write buffer (\"\")"), error in (no error)=w1481) -> (VISA resource name out=w1464:refnum<visa-resource-name>, error out=w1480:errorcluster)  [unwired: 1 out]
        n350 = Insert Into Array(array=w1492, new element=w1513) -> (w1485:dbl[][])  [unwired: 2 in]
        n351 = call <vilib>:"compatOverwrite.vi"("overwrite (F)"=TRUE) -> ("overwrite?"=w1459:T8)
        n352 = Open/Create/Replace File(file path (use dialog)=w1489, error in=w1480, operation (0:open)=w1459) -> (refnum out=w1498:refnum<file>, error out=w1497:errorcluster)  [unwired: 3 in, 1 out]
        n353 = Transpose 2D Array(2D array=w1485) -> (transposed array=w1484:dbl[][])
        n354 = call "4155C Write array to file.vi"("Byte Stream File Refnum"=w1498, "Header"=string[] ["Time /s", "Vdg /V", "Idg /A", "Is /A"], "Data Array"=w1484, "error in (no error)"=w1497) -> ("dup refnum"=w1500:refnum<file>, "error out"=w1499:errorcluster)  [unwired: 1 in]
        n355 = Close File(refnum=w1500, error in=w1499) -> (error out=w1462:errorcluster)  [unwired: 1 out]
        n356 = VISA Write(VISA resource name=w1464, write buffer=";:PAGE:SCON:STAN OFF;:PAGE:CHAN:VSU2:DIS;" ("write buffer (\"\")"), error in (no error)=w1462) -> (VISA resource name out=w1460:refnum<visa-resource-name>, error out=w1461:errorcluster)  [unwired: 1 out]
      }
      frame "#" {
        n357 = VISA Write(VISA resource name=w1540, write buffer=":DISP ON" ("write buffer (\"\")"), error in (no error)=w1539) -> (VISA resource name out=w1538:refnum<visa-resource-name>, error out=w1537:errorcluster)  [unwired: 1 out]
      }
      frame "stressV" {
        n358 = Number To Decimal String(number=w1569) -> (decimal integer string=w1610:string)  [unwired: 1 in]
        n359 = Concatenate Strings(w1594, "-stressV-" ("Substring"), w1610, w1568, ".txt" ("Substring")) -> (w1608:string)
        n360 = Fract/Exp String To Number(string=w1607) -> (number=w1580:dbl[])  [unwired: 3 in, 1 out]
        n361 = String To Path(string=w1608) -> (path=w1598:path)
        n362 = Index Array(array=w1580, index=3 ("Index")) -> (element=w1577:dbl)
        n363 = Index Array(array=w1580, index=1 ("Index")) -> (element=w1575:dbl)
        n364 = Index Array(array=w1580, index=0 ("Index")) -> (element=w1574:dbl)
        n365 = Index Array(array=w1580, index=4 ("Index")) -> (element=w1579:dbl)
        n366 = Index Array(array=w1580, index=2 ("Index")) -> (element=w1576:dbl)
        n367 = call "4155C Config V Stress.vi"("VISA session"=w1613, "ID compliance"=w1577, "VD"=w1575, "VG"=w1574, "IG compliance"=w1576, "error in (no error)"=w1612, "Display on/off"=TRUE) -> ("dup VISA resource name"=w1615:refnum<visa-resource-name>, "error out"=w1614:errorcluster)
        n368 = call "4155C Apply Stress.vi"("error in (no error)"=w1614, "Duration"=w1579, "Emergency Stop"=w1593, "VISA resource name in"=w1615) -> ("error out"=w1591:errorcluster, "VISA Resource Name out"=w1589:refnum<visa-resource-name>)
        n369 = VISA Write(VISA resource name=w1589, write buffer=":DISP ON" ("write buffer (\"\")"), error in (no error)=w1591) -> (VISA resource name out=w1588:refnum<visa-resource-name>, error out=w1590:errorcluster)  [unwired: 1 out]
        n370 = call <vilib>:"compatOverwrite.vi"("overwrite (F)"=TRUE) -> ("overwrite?"=w1573:T8)
        n371 = Open/Create/Replace File(file path (use dialog)=w1598, error in=w1590, operation (0:open)=w1573) -> (refnum out=w1601:refnum<file>, error out=w1600:errorcluster)  [unwired: 3 in, 1 out]
        n372 = call "4155C Write array to file.vi"("Byte Stream File Refnum"=w1601, "Header"=string[] ["V stress completed successfully", ""], "error in (no error)"=w1600) -> ("dup refnum"=w1603:refnum<file>, "error out"=w1602:errorcluster)  [unwired: 2 in]
        n373 = Close File(refnum=w1603, error in=w1602) -> (error out=w1596:errorcluster)  [unwired: 1 out]
      }
      frame "stressI" {
        n374 = Number To Decimal String(number=w1636) -> (decimal integer string=w1673:string)  [unwired: 1 in]
        n375 = Concatenate Strings(w1657, "-stressI-" ("Substring"), w1673, w1635, ".txt" ("Substring")) -> (w1671:string)
        n376 = Fract/Exp String To Number(string=w1670) -> (number=w1645:dbl[])  [unwired: 3 in, 1 out]
        n377 = Index Array(array=w1645, index=1 ("Index")) -> (element=w1641:dbl)
        n378 = Index Array(array=w1645, index=0 ("Index")) -> (element=w1642:dbl)
        n379 = call "4155C Config I Stress.vi"("VISA session"=w1676, "IDG"=w1642, "VDG compliance"=w1641, "error in (no error)"=w1675, "Display on/off"=TRUE) -> ("dup VISA resource name"=w1678:refnum<visa-resource-name>, "error out"=w1677:errorcluster)
        n380 = Index Array(array=w1645, index=2 ("Index")) -> (element=w1643:dbl)
        n381 = String To Path(string=w1671) -> (path=w1661:path)
        n382 = call "4155C Apply Stress.vi"("error in (no error)"=w1677, "Duration"=w1643, "Emergency Stop"=w1656, "VISA resource name in"=w1678) -> ("error out"=w1654:errorcluster, "VISA Resource Name out"=w1652:refnum<visa-resource-name>)
        n383 = VISA Write(VISA resource name=w1652, write buffer=":DISP ON" ("write buffer (\"\")"), error in (no error)=w1654) -> (VISA resource name out=w1651:refnum<visa-resource-name>, error out=w1653:errorcluster)  [unwired: 1 out]
        n384 = call <vilib>:"compatOverwrite.vi"("overwrite (F)"=TRUE) -> ("overwrite?"=w1640:T8)
        n385 = Open/Create/Replace File(file path (use dialog)=w1661, error in=w1653, operation (0:open)=w1640) -> (refnum out=w1664:refnum<file>, error out=w1663:errorcluster)  [unwired: 3 in, 1 out]
        n386 = call "4155C Write array to file.vi"("Byte Stream File Refnum"=w1664, "Header"=string[] ["I stress completed successfully", ""], "error in (no error)"=w1663) -> ("dup refnum"=w1666:refnum<file>, "error out"=w1665:errorcluster)  [unwired: 2 in]
        n387 = Close File(refnum=w1666, error in=w1665) -> (error out=w1659:errorcluster)  [unwired: 1 out]
      }
      frame "vsu2pulse" {
        n388 = Number To Decimal String(number=w1699) -> (decimal integer string=w1734:string)  [unwired: 1 in]
        n389 = Concatenate Strings(w1719, "-vsu2-" ("Substring"), w1734, w1698, ".txt" ("Substring")) -> (w1732:string)
        n390 = Fract/Exp String To Number(string=w1731) -> (number=w1707:dbl[])  [unwired: 3 in, 1 out]
        n391 = String To Path(string=w1732) -> (path=w1723:path)
        n392 = Index Array(array=w1707, index=1 ("Index")) -> (element=w1706:dbl)
        n393 = Index Array(array=w1707, index=0 ("Index")) -> (element=w1704:dbl)
        n394 = call "4155C Config VSU2 Stress.vi"("error in (no error)"=w1736, "VSU2"=w1704, "Display on/off"=TRUE, "VISA session"=w1737) -> ("error out"=w1738:errorcluster, "dup VISA resource name"=w1739:refnum<visa-resource-name>)
        n395 = call "4155C Apply Stress.vi"("error in (no error)"=w1738, "Duration"=w1706, "Emergency Stop"=w1718, "VISA resource name in"=w1739) -> ("error out"=w1716:errorcluster, "VISA Resource Name out"=w1714:refnum<visa-resource-name>)
        n396 = VISA Write(VISA resource name=w1714, write buffer=":DISP ON" ("write buffer (\"\")"), error in (no error)=w1716) -> (VISA resource name out=w1713:refnum<visa-resource-name>, error out=w1715:errorcluster)  [unwired: 1 out]
        n397 = call <vilib>:"compatOverwrite.vi"("overwrite (F)"=TRUE) -> ("overwrite?"=w1703:T8)
        n398 = Open/Create/Replace File(file path (use dialog)=w1723, error in=w1715, operation (0:open)=w1703) -> (refnum out=w1726:refnum<file>, error out=w1725:errorcluster)  [unwired: 3 in, 1 out]
        n399 = call "4155C Write array to file.vi"("Byte Stream File Refnum"=w1726, "Header"=string[] ["VSU2 pulse completed successfully", ""], "error in (no error)"=w1725) -> ("dup refnum"=w1728:refnum<file>, "error out"=w1727:errorcluster)  [unwired: 2 in]
        n400 = Close File(refnum=w1728, error in=w1727) -> (error out=w1721:errorcluster)  [unwired: 1 out]
      }
      frame "sample-fpp" {
        w1771 = string[] ["Time /s", "Id VgVd /A", "Ig VgVd /A", "Vp1 VgVd /V", "Vp2 VgVd /V"] ("Header")
        w1775 = "%d" ("format string")
        n401 = Number To Decimal String(number=w1760) -> (decimal integer string=w1823:string)  [unwired: 1 in]
        n402 = Fract/Exp String To Number(string=w1820) -> (number=w1808:dbl[])  [unwired: 3 in, 1 out]
        n403 = Concatenate Strings(w1814, "-samplefpp-" ("Substring"), w1823, w1759, ".txt" ("Substring")) -> (w1821:string)
        n404 = String To Path(string=w1821) -> (path=w1783:path)
        n405 = Index Array(array=w1808, index=0 ("Index")) -> (element=w1769:dbl)
        n406 = Index Array(array=w1808, index=1 ("Index")) -> (element=w1768:dbl)
        n407 = Index Array(array=w1808, index=2 ("Index")) -> (element=w1816:dbl)
        n408 = Index Array(array=w1808, index=3 ("Index")) -> (element=w1806:dbl)
        n409 = call "4155C Config Sampling Measurements FPP.vi"("VISA session"=w1826, "Num Points"=w1816, "Vg"=w1769, "Display on/off"=TRUE, "Gate Compliance"=w1815, "Drain Compliance"=w1824, "Standby"="Standby", "error in (no error)"=w1825, "Timings"=w1813, "Vd"=w1768, "Sample time"=w1806) -> ("dup VISA resource name"=w1785:refnum<visa-resource-name>, "error out"=w1784:errorcluster)  [unwired: 3 in]
        n410 = Number To Decimal String(number=w1769) -> (decimal integer string=w1795:string)  [unwired: 1 in]
        n411 = call "4155C Take Sample FPP.vi"("VISA resource name in"=w1785, "error in (no error)"=w1784, "Emergency Stop"=w1786) -> ("Time"=w1790:dbl[], "Vp1"=w1800:dbl[], "VISA Resource Name out"=w1766:refnum<visa-resource-name>, "Ig"=w1788:dbl[], "Id"=w1789:dbl[], "Vp2"=w1798:dbl[], "error out"=w1787:errorcluster)  [unwired: 10 in]
        n412 = Insert Into Array(array=dbl[][] [] ("Input Array"), new element=w1790) -> (w1804:dbl[][])  [unwired: 2 in]
        n413 = Number To Decimal String(number=w1768) -> (decimal integer string=w1793:string)  [unwired: 1 in]
        n414 = Insert Into Array(array=w1804, new element=w1789) -> (w1803:dbl[][])  [unwired: 2 in]
        n415 = Concatenate Strings("(Vg = " ("Substring"), w1795, "V, Vd = " ("Substring"), w1793, "V)" ("Substring")) -> (w1791:string)
        n416 = Insert Into Array(array=w1803, new element=w1788) -> (w1802:dbl[][])  [unwired: 2 in]
        n417 = Insert Into Array(array=w1802, new element=w1800) -> (w1799:dbl[][])  [unwired: 2 in]
        n418 = Insert Into Array(array=w1799, new element=w1798) -> (w1767:dbl[][])  [unwired: 2 in]
        n419 = Transpose 2D Array(2D array=w1767) -> (transposed array=w1797:dbl[][])
        n420 = call <vilib>:"compatOverwrite.vi"("overwrite (F)"=TRUE) -> ("overwrite?"=w1764:T8)
        n421 = Open/Create/Replace File(file path (use dialog)=w1783, error in=w1787, operation (0:open)=w1764) -> (refnum out=w1780:refnum<file>, error out=w1781:errorcluster)  [unwired: 3 in, 1 out]
        n422 = Array To Spreadsheet String(array=w1771, 3:w1775) -> (spreadsheet string=w1777:string)  [unwired: 1 in]
        n423 = Search and Replace String(replace all?=TRUE ("replace all? (F)"), input string=w1777, search string="VgVd", replace string=w1791) -> (result string=w1773:string)  [unwired: 4 in, 3 out]
        n424 = Spreadsheet String To Array(format string=w1775, spreadsheet string=w1773, array type (2D Dbl)=w1771) -> (array=w1772:string[])  [unwired: 1 in]
        n425 = call "4155C Write array to file.vi"("Byte Stream File Refnum"=w1780, "Header"=w1772, "Data Array"=w1797, "error in (no error)"=w1781) -> ("dup refnum"=w1778:refnum<file>, "error out"=w1779:errorcluster)  [unwired: 1 in]
        n426 = Close File(refnum=w1778, error in=w1779) -> (error out=w1765:errorcluster)  [unwired: 1 out]
      }
      frame "resample-fpp" {
        w1860 = string[] ["Time /s", "Id VgVd /A", "Ig VgVd /A", "Vp1 VgVd /V", "Vp2 VgVd /V"] ("Header")
        w1864 = "%d" ("format string")
        n427 = Number To Decimal String(number=w1846) -> (decimal integer string=w1904:string)  [unwired: 1 in]
        n428 = Fract/Exp String To Number(string=w1901) -> (number=w1853:dbl[])  [unwired: 3 in, 1 out]
        n429 = Concatenate Strings(w1897, "-resamplefpp-" ("Substring"), w1904, w1847, ".txt" ("Substring")) -> (w1902:string)
        n430 = String To Path(string=w1902) -> (path=w1872:path)
        n431 = Index Array(array=w1853, index=0 ("Index")) -> (element=w1859:dbl)
        n432 = Index Array(array=w1853, index=1 ("Index")) -> (element=w1858:dbl)
        n433 = Number To Decimal String(number=w1859) -> (decimal integer string=w1882:string)  [unwired: 1 in]
        n434 = call "4155C Take Sample FPP.vi"("VISA resource name in"=w1855, "error in (no error)"=w1854, "Emergency Stop"=w1873) -> ("Time"=w1877:dbl[], "Vp1"=w1887:dbl[], "VISA Resource Name out"=w1857:refnum<visa-resource-name>, "Ig"=w1875:dbl[], "Id"=w1876:dbl[], "Vp2"=w1885:dbl[], "error out"=w1874:errorcluster)  [unwired: 10 in]
        n435 = Insert Into Array(array=dbl[][] [] ("Input Array"), new element=w1877) -> (w1891:dbl[][])  [unwired: 2 in]
        n436 = Number To Decimal String(number=w1858) -> (decimal integer string=w1880:string)  [unwired: 1 in]
        n437 = Insert Into Array(array=w1891, new element=w1876) -> (w1890:dbl[][])  [unwired: 2 in]
        n438 = Concatenate Strings("(Vg = " ("Substring"), w1882, "V, Vd = " ("Substring"), w1880, "V)" ("Substring")) -> (w1878:string)
        n439 = Insert Into Array(array=w1890, new element=w1875) -> (w1889:dbl[][])  [unwired: 2 in]
        n440 = Insert Into Array(array=w1889, new element=w1887) -> (w1886:dbl[][])  [unwired: 2 in]
        n441 = Insert Into Array(array=w1886, new element=w1885) -> (w1852:dbl[][])  [unwired: 2 in]
        n442 = call <vilib>:"compatOverwrite.vi"("overwrite (F)"=TRUE) -> ("overwrite?"=w1851:T8)
        n443 = Open/Create/Replace File(file path (use dialog)=w1872, error in=w1874, operation (0:open)=w1851) -> (refnum out=w1869:refnum<file>, error out=w1870:errorcluster)  [unwired: 3 in, 1 out]
        n444 = Array To Spreadsheet String(array=w1860, 3:w1864) -> (spreadsheet string=w1866:string)  [unwired: 1 in]
        n445 = Transpose 2D Array(2D array=w1852) -> (transposed array=w1884:dbl[][])
        n446 = Search and Replace String(replace all?=TRUE ("replace all? (F)"), input string=w1866, search string="VgVd", replace string=w1878) -> (result string=w1862:string)  [unwired: 4 in, 3 out]
        n447 = Spreadsheet String To Array(format string=w1864, spreadsheet string=w1862, array type (2D Dbl)=w1860) -> (array=w1861:string[])  [unwired: 1 in]
        n448 = call "4155C Write array to file.vi"("Byte Stream File Refnum"=w1869, "Header"=w1861, "Data Array"=w1884, "error in (no error)"=w1870) -> ("dup refnum"=w1867:refnum<file>, "error out"=w1868:errorcluster)  [unwired: 1 in]
        n449 = Close File(refnum=w1867, error in=w1868) -> (error out=w1856:errorcluster)  [unwired: 1 out]
      }
      frame "serial" {
        n450 = local read "Termination char\n(0xA = '\\n' = LF)\n(0xD = '\\r' = CR)"() -> (w1932:u8)
        n451 = local read "Enable Termination\nChar (T)"() -> (w1933:bool)
        n452 = Index Array(array=w1940, index=0 ("Index")) -> (element=w1939:string)
        n453 = local read "parity"() -> (w1923:u16)
        n454 = local read "Delay before read (ms)"() -> (w1934:u32)
        n455 = local read "byte count"() -> (w1931:u32)
        n456 = local read "Timeout (ms)"() -> (w1930:u32)
        n457 = local read "VISA resource name"() -> (w1927:refnum<visa-resource-name>)
        n458 = local read "baud rate"() -> (w1926:u32)
        n459 = local read "Serial End Mode for Reads"() -> (w1925:u16)
        n460 = local read "data bits"() -> (w1924:u16)
        n461 = local read "stop bits"() -> (w1929:u16)
        n462 = local read "flow control"() -> (w1928:u16)
        n463 = call "Serial write and read v0.5.vi"("Delay before read (ms)"=w1934, "Termination char\n(0xA = '\\n' = LF)\n(0xD = '\\r' = CR)"=w1932, "Enable Termination\nChar (T)"=w1933, "parity"=w1923, "stop bits"=w1929, "string to write"=w1939, "flow control"=w1928, "byte count"=w1931, "Serial Settings:Serial End Mode for Reads"=w1925, "Timeout (ms)"=w1930, "error in (no error)"=w1945, "VISA resource name"=w1927, "baud rate"=w1926, "data bits"=w1924) -> ("Serial port output"=w1935:string, "error out"=w1944:errorcluster)
        n464 = Build Array (concatenate)(w1935, w1936) -> (w1937:string[])
      }
      frame "pump" {
        # "Time array for valve position"
        # "Time array for absolute plunger position"
        # "Valve position"
        # "Absolute plunger position"
        # "Remove \"_\""
        # "Check if hard stop is pressed."
        # "Check if halt is pressed."
        # "Check if pump is idle. Else halt."
        n465 = Index Array(array=w2010, index=0 ("Index")) -> (element=w1987:string)
        n466 = case shown="\"No error\", Default" w1985 {
          tunnel: w1987 -> [w2046 _ w2048 w2049 w2050 w2051 _ _ w2054 w2055 _]
          tunnel: [w2046 "/1H" w2048 w2049 w2050 w2051 "/1H" "/1H" w2054 w2055 "/1H"] -> w1986
          frame "No error", Default {
          }
          frame "Initialization" {
          }
          frame "Invalid command" {
          }
          frame "Invalid operand" {
          }
          frame "Device not initialized" {
          }
          frame "Internal failure" {
          }
          frame "Plunger overload" {
          }
          frame "Valve overload" {
          }
          frame "Plunger move not allowed" {
          }
          frame "A/D converter failure" {
          }
          frame "Command overflow" {
          }
        }
        n467 = local read "Hard stop pump"() -> (w1989:bool)
        n468 = local read "Halt pump"() -> (w1992:bool)
        n469 = local read "Serial End Mode for Reads"() -> (w1998:u16)
        n470 = local read "flow control"() -> (w2001:u16)
        n471 = local read "stop bits"() -> (w2002:u16)
        n472 = local read "parity"() -> (w1996:u16)
        n473 = local read "Delay before read (ms)"() -> (w2007:u32)
        n474 = local read "byte count"() -> (w2004:u32)
        n475 = local read "Timeout (ms)"() -> (w2003:u32)
        n476 = local read "VISA resource name"() -> (w2000:refnum<visa-resource-name>)
        n477 = local read "baud rate"() -> (w1999:u32)
        n478 = local read "Enable Termination\nChar (T)"() -> (w2006:bool)
        n479 = local read "Termination char\n(0xA = '\\n' = LF)\n(0xD = '\\r' = CR)"() -> (w2005:u8)
        n480 = case shown="True" w1992 {
          tunnel: [w2060 "/1H"] -> w1991
          tunnel: w1986 -> [w2060 _]
          frame False {
          }
          frame True {
            n481 = local write "Halt pump"(FALSE) -> ()
          }
        }
        n482 = case shown="True" w1989 {
          tunnel: [w2057 "/1T"] -> w1990
          tunnel: w1991 -> [w2057 _]
          frame False {
          }
          frame True {
            n483 = local write "Hard stop pump"(FALSE) -> ()
          }
        }
        n484 = local read "data bits"() -> (w1997:u16)
        n485 = String Subset(string=w1981, offset (0)=1) -> (substring=w1979:string)  [unwired: 1 in]
        n486 = call "SPM Pump v0.6.vi"("Termination char\n(0xA = '\\n' = LF)\n(0xD = '\\r' = CR)"=w2005, "Enable Termination\nChar (T)"=w2006, "Timeout (ms)"=w2003, "Serial Settings:Serial End Mode for Reads"=w1998, "byte count"=w2004, "Delay before read (ms)"=w2007, "Time <input>"=w1984, "error in (no error)"=w2015, "Serial port input"=w1990, "VISA resource name"=w2000, "parity"=w1996, "baud rate"=w1999, "stop bits"=w2002, "data bits"=w1997, "flow control"=w2001, "Time units <input>"=w1979) -> ("Input command"=w1978:string, "Serial port data"=w1968:string[], "Pump status"=w1974:string, "Valve position"=w1976:i32, "Absolute plunger position"=w1988:i32, "Serial port"=w1983:string, "error out"=w2014:errorcluster)  [unwired: 1 in, 4 out]
        n487 = case shown="\"?6\"" w1978 {
          tunnel: [w2027 w2035 w2041] -> w1995
          tunnel: w1994 -> [w2027 w2034 w2041]
          tunnel: w1988 -> [_ w2033 _]
          tunnel: w1975 -> [w2026 w2032 w2042]
          tunnel: [w2026 w2032 w2044] -> w1977
          tunnel: w1976 -> [_ _ w2043]
          tunnel: w1973 -> [_ w2031 w2039]
          tunnel: w1972 -> [w2025 w2030 w2040]
          tunnel: [w2025 w2029 w2040] -> w1971
          tunnel: [w2024 w2028 w2038] -> w1970
          tunnel: w1969 -> [w2024 w2028 w2037]
          frame "Q", Default {
          }
          frame "?" {
            n488 = Build Array (concatenate)(w2034, w2033) -> (w2035:i32[])
            n489 = Build Array (concatenate)(w2030, w2031) -> (w2029:i32[])
            n490 = call "4155C Split array.vi"("X data in"=w2029, "Y1 data in"=w2035) -> ("Array of clusters"=w2036:cluster{"Y data in":dbl[], "X data in":dbl[]}[])  [unwired: 5 in, 1 out]
            n491 = local write "Absolute plunger position vs time"(w2036) -> ()
          }
          frame "?6" {
            n492 = Build Array (concatenate)(w2042, w2043) -> (w2044:i32[])
            n493 = Build Array (concatenate)(w2037, w2039) -> (w2038:i32[])
            n494 = call "4155C Split array.vi"("X data in"=w2038, "Y1 data in"=w2044) -> ("Array of clusters"=w2045:cluster{"Y data in":dbl[], "X data in":dbl[]}[])  [unwired: 5 in, 1 out]
            n495 = local write "Valve position vs time"(w2045) -> ()
          }
        }
        n496 = Build Array (concatenate)(w1966, w1968) -> (w1967:string[][])
        n497 = Build Array (concatenate)(w1982, w1983) -> (w2008:string[])
      }
      frame "filename" {
        n498 = Index Array(array=w2064, index=0 ("Index")) -> (element=w2063:string)
      }
    }
    n499 = local read "Time Units"() -> (w69:u16)
    n500 = case shown="2" w69 {
      tunnel: ["Time (Seconds)" ("element") "Time (Minutes)" ("element") "Time (Hours)" ("element")] -> w109
      frame 0 {
      }
      frame 1, Default {
      }
      frame 2 {
      }
    }
    n501 = Build Array(w148, w77, w87, w86, w85, w84, w83, w82, w81, w80, w79, w78, w76) -> (w187:dbl[][])
    n502 = Transpose 2D Array(2D array=w187) -> (transposed array=w186:dbl[][])
    n503 = Concatenate Strings(w128, w71, "Imax_Imin_Ion_Ioff_vs_time.txt" ("Suffix (Imax,Imin,Ion,Ioff)")) -> (w197:string)
    n504 = Build Array(w109, "Is max (A)" ("VAR2 Name"), "Is min (A)" ("VAR2 Name"), "Id max (A)" ("VAR2 Name"), "Id min (A)" ("VAR2 Name"), "Ig max (A)" ("VAR2 Name"), "Ig min (A)" ("VAR2 Name"), "Is on (A)" ("VAR2 Name"), "Is off (A)" ("VAR2 Name"), "Id on (A)" ("VAR2 Name"), "Id off (A)" ("VAR2 Name"), "Ig on (A)" ("VAR2 Name"), "Ig off (A)" ("VAR2 Name")) -> (w192:string[])
    n505 = Array To Spreadsheet String(array=w186, 3:"%e" ("format string")) -> (spreadsheet string=w190:string)  [unwired: 1 in]
    n506 = Array To Spreadsheet String(array=w192, 3:"" ("format string")) -> (spreadsheet string=w191:string)  [unwired: 1 in]
    n507 = String To Path(string=w197) -> (path=w196:path)
    n508 = Build Array(w191, w190) -> (w189:string[])
    n509 = Write to Text File(file (use dialog)=w196, text=w189, error in=w144) -> (refnum out=w198:refnum<file>, error out=w188:errorcluster)  [unwired: 1 in, 1 out]
    n510 = Close File(refnum=w198, error in=w188) -> (error out=w127:errorcluster)  [unwired: 1 out]
    n511 = Build Array(w123, w149) -> (w154:i32[][])
    n512 = Build Array(w109, "Absolute plunger position" ("VAR2 Name")) -> (w157:string[])
    n513 = Transpose 2D Array(2D array=w154) -> (transposed array=w147:i32[][])
    n514 = Array To Spreadsheet String(array=w157, 3:"" ("format string")) -> (spreadsheet string=w156:string)  [unwired: 1 in]
    n515 = Array To Spreadsheet String(array=w147, 3:"%e" ("format string")) -> (spreadsheet string=w153:string)  [unwired: 1 in]
    n516 = Build Array(w156, w153) -> (w159:string[])
    n517 = Concatenate Strings(w128, w71, "plunger_vs_time.txt" ("Suffix (plunger)")) -> (w151:string)
    n518 = String To Path(string=w151) -> (path=w150:path)
    n519 = Write to Text File(file (use dialog)=w150, text=w159, error in=w127) -> (refnum out=w152:refnum<file>, error out=w161:errorcluster)  [unwired: 1 in, 1 out]
    n520 = Close File(refnum=w152, error in=w161) -> (error out=w126:errorcluster)  [unwired: 1 out]
    n521 = Concatenate Strings(w128, w71, "serial_port_output.txt" ("Suffix (serial port log)")) -> (w167:string)
    n522 = String To Path(string=w167) -> (path=w166:path)
    n523 = Build Array(w109, "Serial port input" ("VAR2 Name"), "Pump status" ("VAR2 Name"), "Serial port output: ") -> (w113:string[])
    n524 = Array To Spreadsheet String(array=w119, 3:"" ("format string")) -> (spreadsheet string=w110:string)  [unwired: 1 in]
    n525 = Array To Spreadsheet String(array=w113, 3:"" ("format string")) -> (spreadsheet string=w111:string)  [unwired: 1 in]
    n526 = Array To Spreadsheet String(array=w118, 3:"" ("format string")) -> (spreadsheet string=w172:string)  [unwired: 1 in]
    n527 = Build Array(w111, w110) -> (w112:string[])
    n528 = Write to Text File(file (use dialog)=w166, text=w112, error in=w126) -> (refnum out=w168:refnum<file>, error out=w169:errorcluster)  [unwired: 1 in, 1 out]
    n529 = local write "Serial port data"(w172) -> ()
    n530 = Close File(refnum=w168, error in=w169) -> (error out=w125:errorcluster)  [unwired: 1 out]
    n531 = Build Array(w122, w130) -> (w136:i32[][])
    n532 = Build Array(w109, "Valve port" ("VAR2 Name")) -> (w139:string[])
    n533 = Transpose 2D Array(2D array=w136) -> (transposed array=w131:i32[][])
    n534 = Array To Spreadsheet String(array=w139, 3:"" ("format string")) -> (spreadsheet string=w138:string)  [unwired: 1 in]
    n535 = Array To Spreadsheet String(array=w131, 3:"%e" ("format string")) -> (spreadsheet string=w135:string)  [unwired: 1 in]
    n536 = Build Array(w138, w135) -> (w141:string[])
    n537 = Concatenate Strings(w128, w71, "valve_port_vs_time.txt" ("Suffix (valve)")) -> (w133:string)
    n538 = String To Path(string=w133) -> (path=w132:path)
    n539 = Write to Text File(file (use dialog)=w132, text=w141, error in=w125) -> (refnum out=w134:refnum<file>, error out=w143:errorcluster)  [unwired: 1 in, 1 out]
    n540 = Close File(refnum=w134, error in=w143) -> (error out=w124:errorcluster)  [unwired: 1 out]
  }
  "error out" <- w31
  "Timings Indicator" <- w15
  "Is max" <- w13
  "Id max" <- w13
  "Ig max" <- w13
  "Imax vs time" <- w9
  "I vs Vg" <- w9
  "Imin vs time" <- w9
  "I vs Vd" <- w9
  "Serial port data" <- "" ("Serial port data")
  "Valve position vs time" <- cluster{"Y data in":dbl[], "X data in":dbl[]}[] [] ("Valve position vs time")
  "Is min" <- w12
  "Id min" <- w12
  "Ig min" <- w12
  "Ion vs time" <- w9
  "Ioff vs time" <- w9
  "Is on" <- w11
  "Id on" <- w11
  "Ig on" <- w11
  "Is off" <- w10
  "Id off" <- w10
  "Ig off" <- w10
